vi "UHR-Fleezers Control (fpga) - 11.3h-g.vi"() -> ()   [LabVIEW 2012]
doc: "UHR-Fleezers Instrument Control Code (fpga)"
uses:
  <vilib>/Platform/TimedLoop/XDataNode/timing_clust.ctl
  <vilib>/Platform/TimedLoop/XDataNode/nitl_modes.ctl
  <vilib>/Platform/TimedLoop/XDataNode/wakeup.ctl
  <vilib>/rvi/eio/common/nirviEmuTemplateMethod_errors.vi
  <vilib>/rvi/interface/RandomDataEmulation/nirviRandomDataFPGAFIFO.vi
  <vilib>/rvi/interface/RandomDataEmulation/niFpgaRandomDataHandleErrors.vi
  <vilib>/rvi/Emulation/niFpgaSctlEmulationGetInTimedLoop.vi
  <vilib>/rvi/Emulation/niFpgaSctlEmulationGlobalWrite.vi
  <vilib>/rvi/Emulation/niFpgaSctlEmulationRegisterWithScheduler.vi
  <vilib>/rvi/Emulation/niFpgaSctlEmulationScheduler.vi
  <vilib>/Platform/TimedLoop/XDataNode/XDataNode.xnode
  <vilib>/eio/EIOMethodNode/EIOMethodNode.xnode
  <vilib>/eio/EIONode/EIONode.xnode
  <vilib>/rvi/DataTransferAndStorage/Container/XNode/niFpgaContainer.xnode
  <vilib>/rvi/interface/RandomDataEmulation/nirviRandomDataFpgaReadWriteTemplate.vi
  <vilib>/addons/control/pid/fpga.llb/XNode/niFpgaPID.xnode
  <vilib>/Platform/TimedLoop/XDataNode/XDNodeRunTimeDep.lvlib
panel:
  in  "Tab Control":T1(tab)=enum."Force FB"
  in  "Set 3":bool
  in  "Set 2":bool=TRUE
  in  "Set 1":bool=TRUE
  in  "Trap Pos to FIFO":bool
  in  "N of AI1 Int Acq Sets":i16=2 min=1 max=3 step=1
  out "AI Late Counter":u8
  in  "ai count":u16=400
  in  "+ phase":bool
  in  "Phase count adjustment":i16
  out "Relative phase":i16
  in  "AI to FIFO":bool
  out "BD1 Frequency Out 1":u64
  out "BD1 Frequency Out 2":u64
  out "Trap Pos FIFO Timeout":u16
  out "Trap AI FIFO Timeout":u16
  in  "Trap FIFO Set Timeout":i32
  in  "Tab Control 2":T2(tab)
  in  "RD":bool
  in  "FB1 output high":i16=3000
  in  "FB1 output low":i16
  in  "D1":i16
  in  "I1":i16=5
  in  "P1":i16=10
  in  "Swap F1 and F2":bool
  in  "Cont. Scan":bool
  in  "Abort scan":bool
  in  "Cycles per step":u64
  in  "Scan BD":bool
  in  "Number of scans":u16
  in  "Scan steps":u64
  in  "Scan freq.  increment":i64
  out "Scanning":bool
  in  "Start scan":bool
  in  "OSK Bd 1":bool
  in  "Reset Bd 1":bool
  in  "PMODE":bool
  in  "Direct RF Box \nCommunication":bool
  in  "Data BD 2":u8 format="%08b"
  in  "Data BD 1":u8 format="%08b"
  in  "Address":u8 format="%02x"
  in  "Update Data":bool
  in  "FPGA Controls\n RF Box":bool
  in  "Number Interlace Cycles":u8=2 min=1 max=3
  in  "Interlace Off Parameters":u8=1 min=1 max=3
  in  "Interlace ON/OFF":bool
  out "DIO Relative phase":i16
  in  "Phase count adjustment (DIO)":i16
  in  "+ phase (DIO)":bool
  out "DIO Late Counter":u8
  in  "DIO count 1 (ticks)":u16=400
  in  "DIO count 2 (ticks)":u16=400
  in  "DIO count 3 (ticks)":u16=400
  out "AI2 Y Sum Set 2":i16
  out "AI2 Y Sum Set 1":i16
  in  "FB Setpoint Set 1":i16 min=0 step=1
  in  "FB Reset Set 1":bool
  in  "FB On/Off Set 1":bool
  in  "FB Reset Set 2":bool
  in  "FB On/Off Set 2":bool
  in  "FB Setpoint Set 2":i16 min=0 step=1
  out "Scan I":u64
  in  "Amp switch delay":u16=5
  in  "BD 2 Amplitude 1":u16
  in  "BD 1 Amplitude 1":u16
  in  "BD 2 Frequency 1":u64
  in  "BD 1 Frequency 1":u64
  in  "BD 2 Amplitude 2":u16
  in  "BD 1 Amplitude 2":u16
  in  "BD 2 Frequency 2":u64
  in  "BD 1 Frequency 2":u64
  in  "BD 2 Amplitude 3":u16
  in  "BD 1 Amplitude 3":u16
  in  "BD 2 Frequency 3":u64
  in  "BD 1 Frequency 3":u64
  in  "FB2 output high":fxp<+/-,16,1>=0.999969482421875
  in  "FB2 output low":fxp<+/-,16,1>=-1.0
  in  "P2":fxp<+/-,16,8> format="%.11g"
  in  "I2":fxp<+/-,16,8>=10.0 format="%.11g"
  in  "D2":fxp<+/-,16,8> format="%.11g"
  in  "Negate Diff?":bool
  in  "Diff FB Measurement?":bool
  in  "FB Trig Integrate":u32=1
  out "TTrig?":bool
  in  "TTrig Negate Pos":bool=TRUE
  out "Trap Pos FB Int Signal":fxp<+/-,24,9> format="%.18g"
  out "Trap Pos FB Int-Norm Signal":fxp<+/-,16,1> format="%.16g"
  in  "FPGA TTrig Thresh":i64
  in  "FPGA Trap Trig":bool
  out "Trap Pos FB Action":i64
  in  "Trap Pos. FB Offset Factor":i64
  in  "Trap Pos. FB Mult Factor":i64=2
  in  "Trap Pos. FB Reset":bool
  in  "Trap Pos FB Monitor T1 or T2":bool
  in  "AI1 X Scale":u16
  in  "Trap Pos FB Int Count":u16=100
  in  "Trap Pos FB Negate Action":bool
  out "AI1 X Set 2":fxp<+/-,16,1>
  out "AI1 X Set 1":fxp<+/-,16,1>
  in  "Trap Pos. FB SP":fxp<+/-,16,1>
  in  "Force feedback":bool
  out "TTrig Sig":i64
  out "TTrig Fin Thresh":i64
  in  "1D or 2D Scan?":bool
  in  "Abort scan (MCL)":bool
  in  "MCL Scan Axis":bool
  in  "Cont. Scan (MCL)":bool
  out "Scan I (MCL)":u64
  in  "Number of scans (MCL)":u16
  out "Scanning MCL":bool
  in  "Scan steps (MCL)":u64
  in  "Cycles per step (MCL)":u64
  in  "Scan freq.  increment (MCL)":i16
  in  "Start scan (MCL)":bool
  in  "AO2":i16
  in  "AO1":i16
  out "MCL Late Counter":u8
  in  "MCL count":u32=800
  out "MCL Relative Phase":i16
  in  "Phase count adjustment (MCL)":i16
  in  "+ phase (MCL)":bool
  out "APD3 out state":bool
  in  "APD Gate Operating Mode":u8 max=2 step=1
  in  "Invert APD Gate":bool
  in  "APD Gate OFF Count":u16=100
  in  "APD Gate ON Count":u16=300
  out "APD 1 Gate Late Counter":u8
  out "APD 1 Gate Relative Phase":i16
  in  "Phase count adjustment (APD 1 Gate)":i16
  in  "+ phase (APD 1 Gate)":bool
  out "APD 2 Counts 0":u32
  out "APD 2 Counts 1":u32
  out "APD 1 Counts 0":u32
  out "APD 1 Counts 1":u32
  out "APD1 out state":bool
  in  "APD AO scale factor":i16=1
  in  "APD to FIFO":bool
  in  "APD Acq Rate Count":u32=20000000
  out "APD Acq Late Counter":u8
  out "APD Acq Relative Phase":i16
  in  "Phase Count Adjustment (APD Acq)":i16
  in  "+ phase (APD Acq)":bool
  in  "Phase count adjustment (APD 2 Gate)":i16
  out "APD 2 Gate Late Counter":u8
  out "APD 2 Gate Relative Phase":i16
  in  "+ phase (APD 2 Gate)":bool
  out "APD2 out state":bool
  out "APD 3 Counts 0":u32
  out "APD 3 Counts 1":u32
  out "APD 3 Gate Late Counter":u8
  in  "Phase count adjustment (APD 3 Gate)":i16
  out "APD 3 Gate Relative Phase":i16
  in  "+ phase (APD 3 Gate)":bool
  in  "D3":i16
  in  "I3":i16=5
  in  "P3":i16=10
  in  "Green Filter Flipper":bool
  in  "Green FB Count":u16=1200
  out "Green Late Counter":u8
  out "Green FB Relative Phase":i16
  in  "Phase count adjustment (Green FB)":i16=10
  in  "+ phase (Green FB)":bool
  out "Green FB Sum":i16
  in  "Green int current ON count adj":u16=150
  in  "Current Out":u16=30000
  in  "Green FB On/Off":bool
  in  "Green FB Setpoint":i16=250 min=0 step=1
  in  "Green FB Reset":bool
  in  "Operating Mode 2":u8=2 max=2 step=1
  in  "Invert GI 2":bool
  in  "Green interlace OFF count 2":u16=900
  in  "Green interlace ON count 2":u16=300
  out "GI Late Counter 2":u8
  out "GI Relative phase 2":i16
  in  "Phase count adjustment (GI) 2":i16=20
  in  "+ phase (GI) 2":bool
  in  "Green interlace OFF count":u16=100
  out "GI Relative phase":i16
  in  "Phase count adjustment (GI)":i16
  in  "+ phase (GI)":bool
  in  "Green interlace ON count":u16=300
  out "GI Late Counter":u8
  in  "Invert GI":bool
  in  "Operating Mode":u8 max=2 step=1
  in  "+ phase (RI)":bool
  out "RI Relative phase":i16
  out "RI Late Counter":u8
  in  "Red interlace ON count":u16=300
  in  "Red interlace OFF count":u16=100
  in  "Invert RI":bool
  in  "Red Laser Operating Mode":u8 max=2 step=1
  in  "Phase count adjustment (RI)":i16
  out "Red FB Intensity":i16
  in  "RI Current Out":u16=30000
  in  "Red FB On/Off":bool
  in  "D4":i16
  in  "I4":i16=5
  in  "P4":i16=10
  in  "Red FB Setpoint":i16=250 min=0 step=1
  in  "Red FB Reset":bool
  in  "RI Operating Mode 2":u8=2 max=2 step=1
  in  "Invert RI 2":bool
  in  "Phase count adjustment (BI AO)":i16=20
  in  "Blue current ON count adj (AO)":u16=150
  in  "BI Current Out":i16=30000
  in  "Blue FB On/Off":bool
  in  "D5":i16
  in  "I5":i16=5
  in  "P5":i16=10
  in  "Blue FB Setpoint":i16=250 min=0 step=1
  in  "Blue FB Reset":bool
  in  "BI Operating Mode (AO)":u8=2 max=2 step=1
  in  "Invert BI (AO)":bool
  in  "Blue OFF count (AO)":u16=900
  in  "Blue ON count (AO)":u16=300
  out "BI Late Counter (AO)":u8
  out "BI Relative phase (AO)":i16
  in  "+ phase (BI AO)":bool
  in  "Phase count adjustment (BI D)":i16
  in  "Blue Laser Operating Mode (D)":u8 max=2 step=1
  in  "Invert BI (D)":bool
  in  "Blue interlace OFF count (D)":u16=100
  in  "Blue interlace ON count (D)":u16=300
  out "Blue Late Counter (D)":u8
  out "BI Relative phase (D)":i16
  in  "+ phase (BI D)":bool
  out "Blue Intensity":i16
  # "Only one of these can be on\nat a time:"
  # "Raster Scan AOD"
  # "1 (X)"
  # "2 (Y)"
  # "IR Intensity Feedback (RF BD 1)"
  # "FB Gains Set 1"
  # "FB output range 1"
  # "FB Triggering Excitation Laser"
  # "Trap Pos. FB Gains"
  # "Trap Pos. FB Range"
  # "AO1 (Y)"
  # "2D"
  # "1D"
  # "AO2 (X)"
  # "APD AO for aligning"
  # "Detection Loop"
  # "Green fluorescent laser digital gate interlacing loop"
  # "0 Forced ON\n1 Forced OFF\n2 Interlacing"
  # "Green FB Gains"
  # "Red fluorescent laser digital gate interlacing loop"
  # "Detection Loop"
  # "0 Forced ON\n1 Forced OFF\n2 Interlacing"
  # "Analog/FB Control Loop\n(Disabled)"
  # "Digital Control Loop"
  # "Blue laser intensity reading"
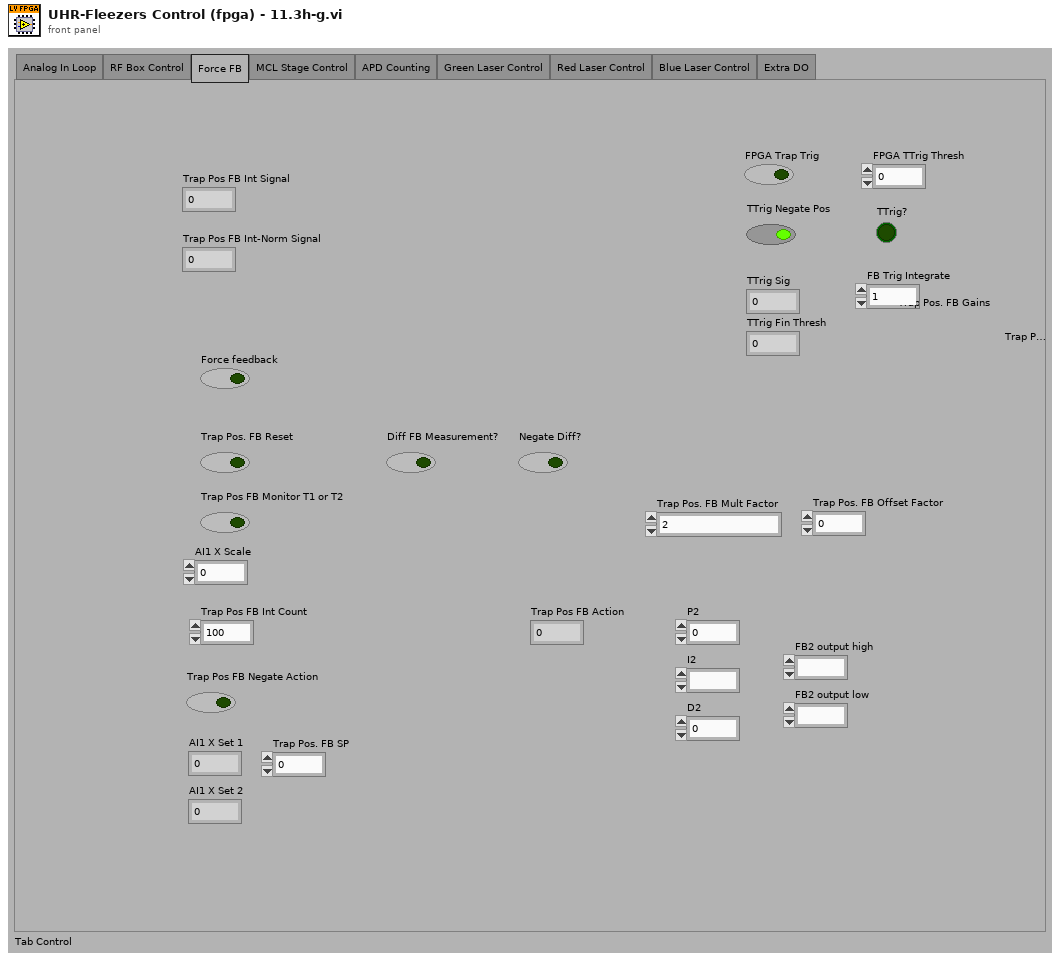
[diagram p1: front panel]
types:
  T1 = enum32{"Analog In Loop", "RF Box Control", "Force FB", "MCL Stage Control", "APD Counting", "Green Laser Control", "Red Laser Control", "Blue Laser Control", "Extra DO"}
  T2 = enum32{"Controls", "Interlacing Frequency and Amplitude Values"}
  T3 = typedef "XDNodeRunTimeDep.lvlib/timing_clust.ctl" = cluster{"Expected End [f-1]":u64, "Actual End [f-1]":u64, "Finished Late? [f-1]":bool, "Expected End [i-1]":u64, "Actual End [i-1]":u64, "Finished Late? [i-1]":bool, "Expected Start [i]":u64, "Actual Start [i]":u64, "Expected Start [f]":u64, "Actual Start [f]":u64, "Source Name":string, "Structure Name":string, "Period":i64, "Deadline":i64, "Offset":i64, "Start":i64, "Priority":i32, "Timeout":i32, "Mode":T4, "Wakeup Reason":T5, "Error":errorcluster, "Source Type":string, "Secondary Source Type":string, "Global End Time":u64, "Global Start Time":u64, "Frame Duration":u64, "Iteration Duration":u64, "Assigned CPU":i32, "I/O Scan Engine Mode":u32}
  T4 = typedef "XDNodeRunTimeDep.lvlib/nitl_modes.ctl" = enum32{"No Change", "Process missed periods, maintain original phase", "Discard missed periods, maintain original phase", "Process missed periods, ignore original phase", "Discard missed periods, ignore original phase"}
  T5 = typedef "XDNodeRunTimeDep.lvlib/wakeup.ctl" = enum32{"Normal", "Aborted", "Asynchronous wakeup", "Timing source error", "Timed loop error", "Timeout"}
  T6 = cluster{"proportional gain (Kc)":i16, "integral gain (Kc*Ts/Ti)":i16, "derivative gain (Kc*Td/Ts)":i16}
  T7 = cluster{"FB1 output high":i16, "FB1 output low":i16}
  T8 = cluster{"P2":fxp<+/-,16,8>, "I2":fxp<+/-,16,8>, "D2":fxp<+/-,16,8>}
  T9 = cluster{"FB2 output high":fxp<+/-,16,1>, "FB2 output low":fxp<+/-,16,1>}
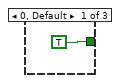
[diagram p3: hidden frame]
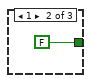
[diagram p4: hidden frame]
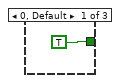
[diagram p5: hidden frame]
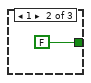
[diagram p6: hidden frame]
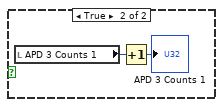
[diagram p7: hidden frame]
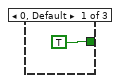
[diagram p8: hidden frame]
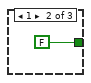
[diagram p9: hidden frame]
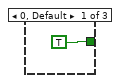
[diagram p10: hidden frame]
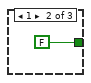
[diagram p11: hidden frame]
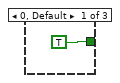
[diagram p12: hidden frame]
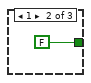
[diagram p13: hidden frame]
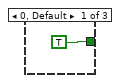
[diagram p14: hidden frame]
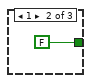
[diagram p15: hidden frame]
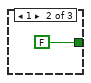
[diagram p18: hidden frame]
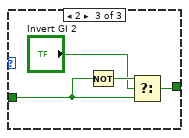
[diagram p19: hidden frame]
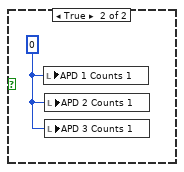
[diagram p20: hidden frame]
diagram:
  w3 = u16 0
  w5 = FALSE
  w2 = FALSE
  # "timing array current index"
  # "timing array"
  # "timing counter (phase adjusted here)"
  # "late counter"
  n1 = flat-sequence "FPGA initialization to do before running any of the loops" {
    tunnel: [u16 0 ("DIO count 3 (ticks)")] -> w1
    tunnel: [w12] -> _
    frame #0 {
      # "Start up expansion chassis early\nto avoid delays later"
      # "This pin controls udclk on the RF boards.\nWhen initially configuring the boards, this pin needs to be\nconfigured as a high impedance input.  Later it will be switched\nto an output."
      # "Initial setting of DIO data and \naddress to low (before reset).  \nThis needs to happen before the other\ncontrol method loops execute."
      n2 = xnode "FPGA I/O Node"("Chassis2/Mod4/AO0"=u16 0) -> ("Chassis2/Mod1/AI0"=w12:i16)  [unwired: 2 in, 2 out]
      n3 = xnode "FPGA I/O Method Node"("Enable"=FALSE) -> ()  [unwired: 1 in, 1 out]
      n4 = xnode "FPGA I/O Node"("Connector1/DIO0"=FALSE, "Connector1/DIO1"=FALSE, "Connector1/DIO2"=FALSE, "Connector1/DIO3"=FALSE, "Connector1/DIO4"=FALSE, "Connector1/DIO5"=FALSE, "Connector1/DIO6"=FALSE, "Connector1/DIO7"=FALSE, "Connector1/DIO8"=FALSE, "Connector1/DIO9"=FALSE, "Connector1/DIO10"=FALSE, "Connector1/DIO11"=FALSE, "Connector1/DIO12"=FALSE, "Connector1/DIO13"=FALSE, "Connector1/DIO15"=FALSE, "Connector1/DIO20"=FALSE, "Connector1/DIO21"=FALSE, "Connector1/DIO22"=FALSE, "Connector1/DIO23"=FALSE, "Connector1/DIO24"=FALSE, "Connector1/DIO25"=FALSE, "Connector1/DIO26"=FALSE, "Connector1/DIO27"=FALSE, "Connector1/DIO14"=FALSE) -> ()  [unwired: 24 in, 24 out]
    }
  }
  n5 = local read "AO1"() -> (w10:i16)
  n6 = local read "AO2"() -> (w9:i16)
  n7 = node-c288() -> (w8:T3)  [unwired: 1 in]
  n8 = timed-loop "RF box board DIO control: control bits" {
    timing: w8 -> [_]
    timing-out: [_] -> w7
    tunnel: [w42] -> _
    tunnel: w1 -> [w42]
    stop <- FALSE stop-if-true
    n9 = xnode "FPGA I/O Node"("Connector1/DIO16"="RD", "Connector1/DIO17"="PMODE", "Connector1/DIO18"="OSK Bd 1", "Connector1/DIO19"="Reset Bd 1", "Connector0/DIO3"="Green Filter Flipper") -> ()  [unwired: 5 in, 5 out]
  }
  n10 = while "RF box board DIO control: parallel communication" {
    shift-right: [w55] -> _
    shift-left: w1 -> [w54]
    shift-right: [w53] -> _
    shift-left: FALSE ("Swap F1 and F2") -> [w52]
    stop <- FALSE stop-if-true
    n11 = flat-sequence {
      tunnel: w52 -> [w59]
      tunnel: w54 -> [w57]
      tunnel: [w59] -> w51
      tunnel: [w58] -> w50
      tunnel: [w57] -> w49
      tunnel: [w65] -> w55
      tunnel: [w64] -> w53
      tunnel: w51 -> [w63]
      tunnel: w50 -> [w61]
      tunnel: w49 -> [w60]
      frame #0 {
        n12 = call "Loop Timer"("Count(Ticks)"=w57) -> ("Tick Count(Ticks)"=w58:u16)
      }
      frame #1 {
        n13 = flat-sequence {
          tunnel: ["FPGA Controls\n RF Box"] -> w62
          tunnel: w63 -> [w66]
          tunnel: [w106] -> w65
          tunnel: [w119] -> w64
          tunnel: w62 -> [w118]
          tunnel: w61 -> [w112]
          tunnel: w60 -> [w109]
          frame #0 {
            n14 = case shown="True" "FPGA Controls\n RF Box" {
              tunnel: w66 -> [_ w68]
              frame False {
              }
              frame True {
                n15 = flat-sequence {
                  tunnel: w68 -> [w74]
                  frame #0 {
                    n16 = First Call?() -> (First Call?: T/F=w69:bool)
                    n17 = case shown="True" w69 {
                      frame False {
                      }
                      frame True {
                        # "If first time data updated, be sure to set WR high and UDCLK low\nbefore setting data and address bits."
                        n18 = xnode "FPGA I/O Method Node"("Enable"=TRUE) -> ("FPGA I/O Out"=w71:refnum<k21>)  [unwired: 1 in]
                        n19 = xnode "FPGA I/O Node"("Connector1/DIO15"=TRUE) -> ()  [unwired: 1 in, 1 out]
                        n20 = xnode "FPGA I/O Node"("I/O Item"=FALSE ("Connector1/DIO30"), "FPGA I/O In"=w71) -> ()  [unwired: 1 out]
                      }
                    }
                  }
                  frame #1 {
                    n21 = flat-sequence {
                      tunnel: w74 -> [w75]
                      frame #0 {
                        # "switch frequency"
                        n22 = xnode "FPGA I/O Node"("Connector1/DIO36"=w75) -> ()  [unwired: 1 in, 1 out]
                      }
                      frame #1 {
                        n23 = call "Wait4"("Count(Ticks)"="Amp switch delay") -> ()  [unwired: 1 out]
                      }
                      frame #2 {
                        # "switch amplitude"
                        # "send udclk high"
                        n24 = xnode "FPGA I/O Node"("Connector1/DIO30"=TRUE ("Connector1/DIO15")) -> ()  [unwired: 1 in, 1 out]
                      }
                      frame #3 {
                        # "send udclk low"
                        n25 = xnode "FPGA I/O Node"("Connector1/DIO30"=FALSE ("Connector1/DIO15")) -> ()  [unwired: 1 in, 1 out]
                      }
                    }
                  }
                }
              }
            }
          }
          frame #1 {
            # "This is the prior cycle's on time"
            # "increment timing\nindex, reset to 0 if \nend of matrix"
            # "Reset to begginning (1) when number of cycles reached."
            # "timing index"
            # "build byte stacks for writing data\n(must correspond to addresses array constant)"
            # "Timing housekeeping"
            # "Adjust phase if late\n(maintains constant phase relationship between cycles)"
            n26 = Bundle("FB1 output high"="FB1 output high", "FB1 output low"="FB1 output low") -> (w79:T7)  [unwired: 1 in]
            n27 = Bundle("P1"="P1", "I1"="I1", "D1"="D1") -> (w80:cluster{"P1":i16, "I1":i16, "D1":i16})  [unwired: 1 in]
            n28 = feedback #1(u8 0 ("t")) -> (w115:u8)
            n29 = Increment(x=w115) -> (x+1=w159:u8)
            n30 = Increment(x="Number Interlace Cycles") -> (x+1=w154:u8)
            n31 = Equal?(x=w159, y=w154) -> (x = y?=w161:bool)
            n32 = Select(t=u8 1, s=w161, f=w159) -> (s? t:f=w114:u8)
            n33 = feedback-in #1(w114) -> ()
            n34 = Increment(x=w114) -> (x+1=w156:u8)
            n35 = Equal?(x=w156, y=w154) -> (x = y?=w157:bool)
            n36 = Select(t=u8 1, s=w157, f=w156) -> (s? t:f=w153:u8)
            n37 = Select(t=w153, s="Interlace ON/OFF", f="Interlace Off Parameters") -> (s? t:f=w137:u8)
            n38 = case shown="1, Default" w137 {
              tunnel: [w233 "BD 1 Frequency 2" "BD 1 Frequency 3"] -> w149
              tunnel: [w232 "BD 2 Frequency 2" "BD 2 Frequency 3"] -> w138
              tunnel: ["BD 2 Amplitude 1" "BD 2 Amplitude 2" "BD 2 Amplitude 3"] -> w94
              tunnel: [w221 w392 "BD 1 Amplitude 3"] -> w97
              tunnel: w80 -> [w195 w389 _]
              tunnel: w79 -> [w196 w388 _]
              frame 1, Default {
                w212 = fxp<+/-,24,9> 0.0 ("AI1 X Set 2")
                w205 = u16 0
                w228 = u64 0 ("f")
                # "This signal integration happens no matter what\nso that correct setpoints can be chosen before \nturning on the FB."
                # "Trap 1"
                n39 = local read "AI1 X Set 2"() -> (w208:fxp<+/-,16,1>)
                n40 = local read "AI1 X Set 1"() -> (w209:fxp<+/-,16,1>)
                n41 = local read "Scanning"() -> (w234:bool)
                n42 = Or(x=w234, y="Start scan") -> (x .or. y?=w226:bool)
                n43 = case shown="False" "Diff FB Measurement?" {
                  tunnel: w208 -> [w242 w251]
                  tunnel: w209 -> [w241 w252]
                  tunnel: [w239 w243] -> w210
                  frame False {
                    n44 = Select(t=w241, s="Trap Pos FB Monitor T1 or T2", f=w242) -> (s? t:f=w239:fxp<+/-,16,1>)
                  }
                  frame True {
                    n45 = Subtract(x=w252, y=w251) -> (x-y=w244:fxp<+/-,17,2>)
                    n46 = Not(x="Negate Diff?") -> (.not. x?=w250:bool)
                    n47 = Boolean To (0,1)(Boolean="Negate Diff?") -> (0, 1=w248:i16)
                    n48 = Boolean To (0,1)(Boolean=w250) -> (0, 1=w249:i16)
                    n49 = Negate(x=w248) -> (-x=w247:i16)
                    n50 = Add(x=w247, y=w249) -> (x+y=w245:i16)
                    n51 = Multiply(x=w245, y=w244) -> (x*y=w243:fxp<+/-,32,17>)
                  }
                }
                n52 = Not(x="Abort scan") -> (.not. x?=w224:bool)
                n53 = And(x=w224, y=w226) -> (x .and. y?=w223:bool)
                n54 = case "For raster scanning" shown="True" w223 {
                  tunnel: [u64 0 w378] -> w229
                  tunnel: "Start scan" -> [_ w363]
                  frame False {
                    n55 = local write "Scanning"(FALSE ("scanning")) -> ()
                  }
                  frame True {
                    w347 = i64 0
                    w346 = u64 0
                    # "scan incr."
                    # "freq. incr. mult."
                    # "count steps"
                    # "count number of cycles"
                    n56 = feedback #2(w346) -> (w375:u64)
                    n57 = Select(t=w346, s=w363, f=w375) -> (s? t:f=w377:u64)
                    n58 = Increment(x=w377) -> (x+1=w374:u64)
                    n59 = Greater?(x="Cycles per step", y=w374) -> (0:w356:bool)
                    n60 = Select(t=w374, s=w356, f=w346) -> (s? t:f=w373:u64)
                    n61 = feedback-in #2(w373) -> ()
                    n62 = feedback #3(w346) -> (w372:u64)
                    n63 = Select(t=w346, s=w363, f=w372) -> (s? t:f=w367:u64)
                    n64 = Increment(x=w367) -> (x+1=w371:u64)
                    n65 = Add(x="Scan steps", y="Scan steps") -> (x+y=w370:u64)
                    n66 = Select(t=w367, s=w356, f=w371) -> (s? t:f=w351:u64)
                    n67 = Greater?(x=w370, y=w351) -> (0:w350:bool)
                    n68 = Select(t=w351, s=w350, f=w346) -> (s? t:f=w368:u64)
                    n69 = feedback-in #3(w368) -> ()
                    n70 = Equal?(x="Scan steps", y=w351) -> (x = y?=w355:bool)
                    n71 = Greater?(x="Scan steps", y=w367) -> (0:w366:bool)
                    n72 = feedback #4(w347) -> (w369:i64)
                    n73 = Select(t=w347, s=w363, f=w369) -> (s? t:f=w353:i64)
                    n74 = Increment(x=w353) -> (x+1=w365:i64)
                    n75 = Decrement(x=w353) -> (x-1=w364:i64)
                    n76 = Select(t=w365, s=w366, f=w364) -> (s? t:f=w354:i64)
                    n77 = Select(t=w353, s=w355, f=w354) -> (s? t:f=w352:i64)
                    n78 = Select(t=w353, s=w356, f=w352) -> (s? t:f=w348:i64)
                    n79 = Select(t=w348, s=w350, f=w347) -> (s? t:f=w349:i64)
                    n80 = feedback-in #4(w349) -> ()
                    n81 = feedback #5(w346) -> (w362:u64)
                    n82 = Select(t=w346, s=w363, f=w362) -> (s? t:f=w358:u64)
                    n83 = Increment(x=w358) -> (x+1=w359:u64)
                    n84 = Select(t=w358, s=w350, f=w359) -> (s? t:f=w357:u64)
                    n85 = Greater?(x="Number of scans", y=w357) -> (0:w343:bool)
                    n86 = Multiply(x="Scan freq.  increment", y=w353) -> (x*y=w378:i64)
                    n87 = Select(t=TRUE, s="Cont. Scan", f=w343) -> (s? t:f=w342:bool)
                    "Scanning" <- w342
                    n88 = Select(t=w357, s=w342, f=w346) -> (s? t:f=w360:u64)
                    n89 = feedback-in #5(w360) -> ()
                    n90 = Increment(x=w357) -> (x+1=→"Scan I":u64)
                  }
                }
                n91 = feedback #6(w205) -> (w204:u16)
                n92 = Increment(x=w204) -> (x+1=w206:u16)
                n93 = Greater Or Equal?(x=w206, y="Trap Pos FB Int Count") -> (x >= y?=w197:bool)
                n94 = Select(t=w205, s=w197, f=w206) -> (s? t:f=w207:u16)
                n95 = feedback-in #6(w207) -> ()
                n96 = feedback #7(w212) -> (w211:fxp<+/-,24,9>)
                n97 = Add(x=w210, y=w211) -> (x+y=w203:fxp<+/-,24,9>)
                n98 = case "For intensity feedback" shown="True" "FB On/Off Set 1" {
                  tunnel: "BD 1 Amplitude 1" -> [w380 _]
                  tunnel: [w380 w384] -> w221
                  tunnel: w196 -> [_ w381]
                  tunnel: w195 -> [_ w382]
                  frame False {
                  }
                  frame True {
                    n99 = local read "AI2 Y Sum Set 1"() -> (w385:i16)
                    n100 = call "Slower PID.vi"("process variable"=w385, "reset?"="FB Reset Set 1", "setpoint"="FB Setpoint Set 1", "PID gains (x 2^8)"=w382, "output range"=w381) -> ("output"=w386:i16)  [unwired: 10 out]
                    n101 = To Unsigned Word Integer(number=w386) -> (unsigned 16bit integer=w384:u16)
                  }
                }
                n102 = Select(t=w212, s=w197, f=w203) -> (s? t:f=w215:fxp<+/-,24,9>)
                n103 = feedback-in #7(w215) -> ()
                n104 = Divide(x=w203, y="Trap Pos FB Int Count") -> (x/y=w198:fxp<+/-,16,1>)
                n105 = feedback #8(fxp<+/-,24,9> 0.0 ("AI1 X Set 2")) -> (w216:fxp<+/-,24,9>)
                n106 = Select(t=w203, s=w197, f=w216) -> (s? t:f=w217:fxp<+/-,24,9>)
                "Trap Pos FB Int Signal" <- w217
                n107 = feedback-in #8(w217) -> ()
                n108 = feedback #9(fxp<+/-,16,1> 0.0 ("Trap Pos FB Int-Norm Signal")) -> (w200:fxp<+/-,16,1>)
                n109 = Select(t=w198, s=w197, f=w200) -> (s? t:f=w199:fxp<+/-,16,1>)
                "Trap Pos FB Int-Norm Signal" <- w199
                n110 = feedback-in #9(w199) -> ()
                n111 = case "For position feedback" shown="True" "Force feedback" {
                  tunnel: [i64 0 w258] -> w218
                  tunnel: w198 -> [_ w255]
                  tunnel: w197 -> [_ w254]
                  frame False {
                  }
                  frame True {
                    n112 = feedback #10(i64 0) -> (w257:i64)
                    n113 = case shown="True" w254 {
                      tunnel: [w259 w273] -> w258
                      tunnel: w257 -> [w259 _]
                      tunnel: w255 -> [_ w267]
                      frame False {
                      }
                      frame True {
                        w277 = u32 0
                        n114 = Bundle("P2"="P2", "I2"="I2", "D2"="D2") -> (w263:T8)  [unwired: 1 in]
                        n115 = Bundle("FB2 output high"="FB2 output high", "FB2 output low"="FB2 output low") -> (w260:T9)  [unwired: 1 in]
                        n116 = xnode ("PID")("process variable"=w267, "reset?"="Trap Pos. FB Reset", "setpoint"="Trap Pos. FB SP", "PID gains"=w263, "output range"=w260) -> ("output"=w289:fxp<+/-,16,1>)
                        n117 = Negate(x=w289) -> (-x=w288:fxp<+/-,17,2>)
                        n118 = Select(t=w288, s="Trap Pos FB Negate Action", f=w289) -> (s? t:f=w285:fxp<+/-,17,2>)
                        n119 = Scale By Power Of 2(n=u32 15, x=u32 1) -> (x*2^n=w282:u32)
                        n120 = Multiply(x=w285, y=w282) -> (x*y=w281:fxp<+/-,17,17>)
                        n121 = To Quad Integer(1:w281) -> (0:w293:i64)
                        "Trap Pos FB Action" <- w293
                        n122 = Multiply(x=w293, y="Trap Pos. FB Mult Factor") -> (x*y=w291:i64)
                        n123 = Add(x=w291, y="Trap Pos. FB Offset Factor") -> (x+y=w273:i64)
                        n124 = feedback #11() -> (w274:i64)  [unwired: 1 in]
                        n125 = Add(x=w273, y=w274) -> (x+y=w271:i64)
                        n126 = feedback #12(w277) -> (w279:u32)
                        n127 = Increment(x=w279) -> (x+1=w268:u32)
                        n128 = Greater Or Equal?(x=w268, y="FB Trig Integrate") -> (x >= y?=w269:bool)
                        n129 = Select(t=i64 0, s=w269, f=w271) -> (s? t:f=w275:i64)
                        n130 = feedback-in #11(w275) -> ()
                        n131 = Select(t=w277, s=w269, f=w268) -> (s? t:f=w278:u32)
                        n132 = feedback-in #12(w278) -> ()
                        n133 = And(x=w269, y="FPGA Trap Trig") -> (x .and. y?=w276:bool)
                        n134 = case "Trap FB trigger excitation laser ON" shown="True" w276 {
                          tunnel: w271 -> [_ w297]
                          tunnel: w268 -> [_ w295]
                          frame False {
                          }
                          frame True {
                            n135 = Not(x="TTrig Negate Pos") -> (.not. x?=w304:bool)
                            n136 = Boolean To (0,1)(Boolean="TTrig Negate Pos") -> (0, 1=w302:i16)
                            n137 = Boolean To (0,1)(Boolean=w304) -> (0, 1=w303:i16)
                            n138 = Negate(x=w302) -> (-x=w301:i16)
                            n139 = Add(x=w301, y=w303) -> (x+y=w300:i16)
                            n140 = Multiply(x=w300, y=w297) -> (x*y=w299:i64)
                            "TTrig Sig" <- w299
                            n141 = Multiply(x="FPGA TTrig Thresh", y=w295) -> (x*y=w296:i64)
                            "TTrig Fin Thresh" <- w296
                            n142 = Greater Or Equal?(x=w299, y=w296) -> (x >= y?=w298:bool)
                            n143 = case shown="True" w298 {
                              frame False {
                              }
                              frame True {
                                w307 = TRUE ("Green FB On/Off")
                                w309 = u8 2 ("Operating Mode")
                                n144 = local write "Operating Mode 2"(w309) -> ()
                                n145 = local write "Operating Mode"(w309) -> ()
                                n146 = local write "Green FB On/Off"(w307) -> ()
                                n147 = local write "FPGA Trap Trig"(FALSE ("FPGA Trap Trig")) -> ()
                                "TTrig?" <- w307
                              }
                            }
                          }
                        }
                      }
                    }
                    n148 = feedback-in #10(w258) -> ()
                  }
                }
                n149 = Select(t=w228, s="Scan BD", f=w229) -> (s? t:f=w227:u64)
                n150 = Select(t=w229, s="Scan BD", f=w228) -> (s? t:f=w230:u64)
                n151 = Add(x=w227, y="BD 2 Frequency 1") -> (x+y=w232:u64)
                n152 = Compound Arithmetic op=ADD("BD 1 Frequency 1", w218, w230) -> (w233:u64)
                "BD1 Frequency Out 1" <- w233
              }
              frame 2 {
                # "Trap 2"
                n153 = case shown="True" "FB On/Off Set 2" {
                  tunnel: [w396 w399] -> w392
                  tunnel: "BD 1 Amplitude 2" -> [w396 _]
                  tunnel: w389 -> [_ w398]
                  tunnel: w388 -> [_ w397]
                  frame False {
                  }
                  frame True {
                    n154 = local read "AI2 Y Sum Set 2"() -> (w402:i16)
                    n155 = call "Slower PID.vi"("process variable"=w402, "reset?"="FB Reset Set 2", "setpoint"="FB Setpoint Set 2", "PID gains (x 2^8)"=w398, "output range"=w397) -> ("output"=w400:i16)  [unwired: 10 out]
                    n156 = To Unsigned Word Integer(number=w400) -> (unsigned 16bit integer=w399:u16)
                  }
                }
                "BD1 Frequency Out 2" <- "BD 1 Frequency 2"
              }
              frame 3 {
                # "Fluorescence period"
              }
            }
            n157 = feedback-in #13(w112) -> ()
            n158 = feedback #13(w112) -> (w111:u16)
            n159 = Select(t=w114, s="Interlace ON/OFF", f="Interlace Off Parameters") -> (s? t:f=w152:u8)
            n160 = Subtract(x=w112, y=w111) -> (x-y=w110:u16)
            n161 = Subtract "The error"(x=w110, y=w109) -> (x-y=w87:u16)
            n162 = case shown="1, Default" w152 {
              tunnel: ["DIO count 1 (ticks)" "DIO count 2 (ticks)" "DIO count 3 (ticks)"] -> w108
              frame 1, Default {
              }
              frame 2 {
              }
              frame 3 {
              }
            }
            n163 = Number To Boolean Array(number=w87) -> (Boolean array=w88:bool[])
            n164 = Or Array Elements(Boolean array=w88) -> (logical OR=w86:bool)
            n165 = Boolean To (0,1)(Boolean=w86) -> (0, 1=w93:i16)
            n166 = To Unsigned Byte Integer(number=w93) -> (unsigned 8bit integer=w90:u8)
            n167 = feedback #14(u8 0) -> (w91:u8)
            n168 = Add(x=w90, y=w91) -> (x+y=w89:u8)
            "DIO Late Counter" <- w89
            n169 = feedback-in #14(w89) -> ()
            n170 = Subtract(x=w108, y=w87) -> (x-y=w107:u16)
            n171 = Split Number(x=w149) -> (hi(x)=w148:u32, lo(x)=w147:u32)
            n172 = Split Number(x=w138) -> (hi(x)=w143:u32, lo(x)=w142:u32)
            n173 = Boolean To (0,1)(Boolean="+ phase (DIO)") -> (0, 1=w104:i16)
            n174 = Split Number(x=w148) -> (lo(x)=w146:u16)  [unwired: 1 out]
            n175 = Split Number(x=w147) -> (hi(x)=w145:u16, lo(x)=w144:u16)
            n176 = Split Number(x=w143) -> (lo(x)=w141:u16)  [unwired: 1 out]
            n177 = Split Number(x=w142) -> (hi(x)=w140:u16, lo(x)=w139:u16)
            n178 = Split Number(x=w97) -> (hi(x)=w99:u8, lo(x)=w98:u8)
            n179 = Split Number(x=w94) -> (hi(x)=w96:u8, lo(x)=w95:u8)
            n180 = Split Number(x=w146) -> (hi(x)=w136:u8, lo(x)=w135:u8)
            n181 = Split Number(x=w145) -> (hi(x)=w134:u8, lo(x)=w133:u8)
            n182 = Split Number(x=w141) -> (hi(x)=w129:u8, lo(x)=w128:u8)
            n183 = Split Number(x=w144) -> (hi(x)=w132:u8, lo(x)=w131:u8)
            n184 = Split Number(x=w140) -> (hi(x)=w127:u8, lo(x)=w126:u8)
            n185 = Split Number(x=w139) -> (hi(x)=w125:u8, lo(x)=w124:u8)
            n186 = Multiply(x=w104, y="Phase count adjustment (DIO)") -> (x*y=w100:i16)
            n187 = feedback #15(i16 0) -> (w102:i16)
            n188 = Subtract(x=w102, y=w100) -> (x-y=w101:i16)
            "DIO Relative phase" <- w101
            n189 = feedback-in #15(w101) -> ()
            n190 = Add(x=w107, y=w100) -> (x+y=w106:u16)
            n191 = Build Array "BD 1 A Stack"(w99, w98) -> (w121:u8[])
            n192 = Build Array "BD 2 A Stack"(w96, w95) -> (w120:u8[])
            n193 = Build Array "BD 1 nu Stack"(w136, w135, w134, w133, w132, w131) -> (w130:u8[])
            n194 = Build Array "BD 2 nu Stack"(w129, w128, w127, w126, w125, w124) -> (w123:u8[])
            n195 = case shown="2" w137 {
              tunnel: [w187 w190] -> w119
              tunnel: [u8 10 u8 4] -> w122
              tunnel: "Swap F1 and F2" -> [w188 w190]
              frame 2 {
                # "F2"
                n196 = Not(x=w188) -> (.not. x?=w187:bool)
              }
              frame 1, Default {
                # "low chooses F1"
                # "F1"
              }
            }
            n197 = case "If FPGA is controlling (toggling) RF synth" shown="True" w118 {
              tunnel: w130 -> [_ w166]
              tunnel: w123 -> [_ w165]
              tunnel: w122 -> [_ w164]
              tunnel: w121 -> [_ w163]
              tunnel: w120 -> [_ w162]
              frame False {
              }
              frame True {
                # "Write next amp.\n(wait until beginning of next loop iteration to update)"
                n198 = flat-sequence "Update the next F1 and F2 frequency value (the actual frequency won't change until FSK is switched).\nThen load the next amplitude value into buffer, but don't update it until the next cycle." {
                  tunnel: w166 -> [w169]
                  tunnel: w165 -> [w168]
                  tunnel: w164 -> [w167]
                  tunnel: w163 -> [w180]
                  tunnel: w162 -> [w179]
                  frame #0 {
                    n199 = for {
                      tunnel: w169 -> [w175] mode=indexing
                      tunnel: w168 -> [w174] mode=indexing
                      tunnel: w167 -> [w172]
                      i -> [w173]
                      # "Write next freq."
                      n200 = To Unsigned Byte Integer(number=w173) -> (unsigned 8bit integer=w170:u8)
                      n201 = Add(x=w172, y=w170) -> (x+y=w171:u8)
                      n202 = call "write to RF synth bd.vi"("Address Byte"=w171, "BD 2 Byte"=w174, "BD 1 Byte"=w175) -> ()
                    }
                  }
                  frame #1 {
                    # "send udclk high"
                    n203 = xnode "FPGA I/O Node"("Connector1/DIO30"=TRUE ("Connector1/DIO15")) -> ()  [unwired: 1 in, 1 out]
                  }
                  frame #2 {
                    n204 = xnode "FPGA I/O Node"("Connector1/DIO30"=FALSE ("Connector1/DIO15")) -> ()  [unwired: 1 in, 1 out]
                  }
                  frame #3 {
                    n205 = for {
                      tunnel: w180 -> [w186] mode=indexing
                      tunnel: w179 -> [w185] mode=indexing
                      tunnel: u8 33 -> [w183]
                      i -> [w184]
                      n206 = To Unsigned Byte Integer(number=w184) -> (unsigned 8bit integer=w181:u8)
                      n207 = Add(x=w183, y=w181) -> (x+y=w182:u8)
                      n208 = call "write to RF synth bd.vi"("Address Byte"=w182, "BD 2 Byte"=w185, "BD 1 Byte"=w186) -> ()
                    }
                  }
                }
              }
            }
          }
        }
      }
    }
  }
  n209 = while "RF box board direct communication loop" {
    tunnel: w1 -> [_]
    stop <- FALSE stop-if-true
    n210 = case "Whether to use direct communication method (only use one method at a time)" shown="True" "Direct RF Box \nCommunication" {
      frame False {
      }
      frame True {
        n211 = case shown="True" "Update Data" {
          frame False {
          }
          frame True {
            n212 = flat-sequence {
              frame #0 {
                n213 = First Call?() -> (First Call?: T/F=w411:bool)
                n214 = case shown="True" w411 {
                  frame False {
                  }
                  frame True {
                    # "If first time data updated, be sure to set WR high\nbefore setting data and address bits."
                    n215 = flat-sequence {
                      frame #0 {
                        n216 = xnode "FPGA I/O Node"("Connector1/DIO15"=TRUE) -> ()  [unwired: 1 in, 1 out]
                      }
                      frame #1 {
                        n217 = call "Wait"("Count(Ticks)"=u8 40 ("DO Delay 3 (Ticks)")) -> ()  [unwired: 1 out]
                      }
                    }
                  }
                }
              }
              frame #1 {
                n218 = Number To Boolean Array(number="Address") -> (Boolean array=w460:bool[])
                n219 = Number To Boolean Array(number="Data BD 1") -> (Boolean array=w461:bool[])
                n220 = Number To Boolean Array(number="Data BD 2") -> (Boolean array=w430:bool[])
                n221 = Index Array(array=w461, index=7) -> (element=w445:bool)
                n222 = Index Array(array=w461, index=6) -> (element=w444:bool)
                n223 = Index Array(array=w461, index=5) -> (element=w443:bool)
                n224 = Index Array(array=w461, index=4) -> (element=w442:bool)
                n225 = Index Array(array=w461, index=3) -> (element=w441:bool)
                n226 = Index Array(array=w461, index=2) -> (element=w440:bool)
                n227 = Index Array(array=w461, index=1) -> (element=w439:bool)
                n228 = Index Array(array=w461, index=0) -> (element=w438:bool)
                n229 = Index Array(array=w460, index=5) -> (element=w437:bool)
                n230 = Index Array(array=w460, index=4) -> (element=w436:bool)
                n231 = Index Array(array=w460, index=3) -> (element=w435:bool)
                n232 = Index Array(array=w460, index=2) -> (element=w434:bool)
                n233 = Index Array(array=w460, index=1) -> (element=w433:bool)
                n234 = Index Array(array=w460, index=0) -> (element=w432:bool)
                n235 = Index Array(array=w430, index=7) -> (element=w421:bool)
                n236 = Index Array(array=w430, index=6) -> (element=w420:bool)
                n237 = Index Array(array=w430, index=5) -> (element=w419:bool)
                n238 = Index Array(array=w430, index=4) -> (element=w418:bool)
                n239 = Index Array(array=w430, index=3) -> (element=w417:bool)
                n240 = Index Array(array=w430, index=2) -> (element=w416:bool)
                n241 = Index Array(array=w430, index=1) -> (element=w415:bool)
                n242 = Index Array(array=w430, index=0) -> (element=w414:bool)
                n243 = xnode "FPGA I/O Node"("Connector1/DIO0"=w445, "Connector1/DIO1"=w444, "Connector1/DIO2"=w443, "Connector1/DIO3"=w442, "Connector1/DIO4"=w441, "Connector1/DIO5"=w440, "Connector1/DIO6"=w439, "Connector1/DIO7"=w438, "Connector1/DIO8"=w437, "Connector1/DIO9"=w436, "Connector1/DIO10"=w435, "Connector1/DIO11"=w434, "Connector1/DIO12"=w433, "Connector1/DIO13"=w432, "Connector1/DIO20"=w421, "Connector1/DIO21"=w420, "Connector1/DIO22"=w419, "Connector1/DIO23"=w418, "Connector1/DIO24"=w417, "Connector1/DIO25"=w416, "Connector1/DIO26"=w415, "Connector1/DIO27"=w414) -> ()  [unwired: 22 in, 22 out]
              }
              frame #2 {
                # "wait and then apply write signal"
                n244 = call "Wait2"("Count(Ticks)"=u8 40 ("DO Delay 1 (Ticks)")) -> ()  [unwired: 1 out]
              }
              frame #3 {
                # "sending bit low writes data to board buffer"
                n245 = xnode "FPGA I/O Node"("Connector1/DIO15"=FALSE) -> ()  [unwired: 1 in, 1 out]
              }
              frame #4 {
                # "wait then return write signal"
                n246 = call "Wait3"("Count(Ticks)"=u8 40 ("DO Delay 2 (Ticks)")) -> ()  [unwired: 1 out]
              }
              frame #5 {
                # "sending bit high makes ready to\nwrite more data"
                n247 = xnode "FPGA I/O Node"("Connector1/DIO15"=TRUE) -> ()  [unwired: 1 in, 1 out]
              }
            }
          }
        }
      }
    }
  }
  n248 = To Unsigned Long Integer(number=w1) -> (unsigned 32bit integer=w6:u32)
  n249 = while "APD 1 Counter" {
    tunnel: w1 -> [_]
    stop <- FALSE stop-if-true
    n250 = flat-sequence {
      frame #0 {
        n251 = xnode "FPGA I/O Method Node"("FPGA I/O In"=refnum<k21> "Connector0/DIO0" ("APD 1 DO"), "Timeout"=-1) -> ()  [unwired: 2 out]
      }
      frame #1 {
        n252 = local read "APD1 out state"() -> (w471:bool)
        n253 = case shown="False" w471 {
          frame False {
            n254 = local read "APD 1 Counts 0"() -> (w473:u32)
            n255 = Increment(x=w473) -> (x+1=→"APD 1 Counts 0":u32)
          }
          frame True {
            n256 = local read "APD 1 Counts 1"() -> (w475:u32)
            n257 = Increment(x=w475) -> (x+1=→"APD 1 Counts 1":u32)
          }
        }
      }
    }
  }
  n258 = while "APD 2 Counter" {
    tunnel: w1 -> [_]
    stop <- FALSE stop-if-true
    n259 = flat-sequence {
      frame #0 {
        n260 = xnode "FPGA I/O Method Node"("FPGA I/O In"=refnum<k21> "Connector0/DIO1" ("APD 2 DO"), "Timeout"=-1) -> ()  [unwired: 2 out]
      }
      frame #1 {
        n261 = local read "APD2 out state"() -> (w479:bool)
        n262 = case shown="False" w479 {
          frame False {
            n263 = local read "APD 2 Counts 0"() -> (w481:u32)
            n264 = Increment(x=w481) -> (x+1=→"APD 2 Counts 0":u32)
          }
          frame True {
            n265 = local read "APD 2 Counts 1"() -> (w483:u32)
            n266 = Increment(x=w483) -> (x+1=→"APD 2 Counts 1":u32)
          }
        }
      }
    }
  }
  n267 = while "APD 2 Gating" {
    shift-right: [w487] -> _
    shift-left: w1 -> [w492]
    shift-right: [w486] -> _
    shift-left: w5 -> [w484]
    stop <- FALSE stop-if-true
    n268 = flat-sequence {
      tunnel: w492 -> [w495]
      tunnel: [w496] -> w490
      tunnel: [w495] -> w488
      tunnel: [w494] -> w485
      tunnel: w484 -> [w494]
      tunnel: [w499] -> w491
      tunnel: w490 -> [w499]
      tunnel: [w498] -> w489
      tunnel: w488 -> [w498]
      tunnel: w485 -> [w497]
      tunnel: [w517] -> w487
      tunnel: w491 -> [w528]
      tunnel: w489 -> [w526]
      tunnel: [w521] -> w486
      frame #0 {
        n269 = call "Loop Timer8"("Count(Ticks)"=w495) -> ("Tick Count(Ticks)"=w496:u16)
      }
      frame #1 {
        # "Signal is then sent through \na transistor before APD"
        n270 = xnode "FPGA I/O Node"("Connector0/DIO8"=w497) -> ()  [unwired: 1 in, 1 out]
      }
      frame #2 {
        n271 = local read "APD Gate ON Count"() -> (w510:u16)
        n272 = local read "APD Gate OFF Count"() -> (w509:u16)
        n273 = feedback #16(TRUE) -> (w523:bool)
        n274 = feedback-in #17(w528) -> ()
        n275 = feedback #17(w528) -> (w511:u16)
        n276 = Not(x=w523) -> (.not. x?=w520:bool)
        n277 = feedback-in #16(w520) -> ()
        n278 = Subtract(x=w528, y=w511) -> (x-y=w527:u16)
        n279 = Select(t=w510, s=w520, f=w509) -> (s? t:f=w525:u16)
        n280 = Subtract(x=w527, y=w526) -> (x-y=w502:u16)
        n281 = Subtract(x=w525, y=w502) -> (x-y=w516:u16)
        n282 = Number To Boolean Array(number=w502) -> (Boolean array=w501:bool[])
        n283 = Or Array Elements(Boolean array=w501) -> (logical OR=w500:bool)
        n284 = Boolean To (0,1)(Boolean="+ phase (APD 2 Gate)") -> (0, 1=w514:i16)
        n285 = Multiply(x=w514, y="Phase count adjustment (APD 2 Gate)") -> (x*y=w512:i16)
        n286 = Boolean To (0,1)(Boolean=w500) -> (0, 1=w507:i16)
        n287 = Add(x=w516, y=w512) -> (x+y=w517:u16)
        n288 = To Unsigned Byte Integer(number=w507) -> (unsigned 8bit integer=w504:u8)
        n289 = feedback #18(i16 0) -> (w519:i16)
        n290 = Subtract(x=w519, y=w512) -> (x-y=w518:i16)
        "APD 2 Gate Relative Phase" <- w518
        n291 = feedback-in #18(w518) -> ()
        n292 = feedback #19(u8 0) -> (w505:u8)
        n293 = Add(x=w504, y=w505) -> (x+y=w503:u8)
        "APD 2 Gate Late Counter" <- w503
        n294 = feedback-in #19(w503) -> ()
        n295 = local read "APD Gate Operating Mode"() -> (w508:u8)
        n296 = case shown="2" w508 {
          tunnel: [TRUE FALSE w534] -> w521
          tunnel: w523 -> [_ _ w532]
          frame 0, Default {
          }
          frame 1 {
          }
          frame 2 {
            n297 = local read "Invert APD Gate"() -> (w531:bool)
            n298 = Not(x=w532) -> (.not. x?=w533:bool)
            n299 = Select(t=w533, s=w531, f=w532) -> (s? t:f=w534:bool)
          }
        }
      }
    }
  }
  n300 = while "532 nm green fluorescent laser interlacing (DO to IA 532 nm AOM ME amp)." {
    shift-right: [w538] -> _
    shift-left: w1 -> [w543]
    shift-right: [w537] -> _
    shift-left: w2 -> [w535]
    stop <- FALSE stop-if-true
    n301 = flat-sequence {
      tunnel: w543 -> [w546]
      tunnel: [w547] -> w541
      tunnel: [w546] -> w539
      tunnel: [w545] -> w536
      tunnel: w535 -> [w545]
      tunnel: [w550] -> w542
      tunnel: w541 -> [w550]
      tunnel: [w549] -> w540
      tunnel: w539 -> [w549]
      tunnel: w536 -> [w548]
      tunnel: [w559] -> w538
      tunnel: w542 -> [w579]
      tunnel: w540 -> [w576]
      tunnel: [w568] -> w537
      frame #0 {
        n302 = call "Loop Timer4"("Count(Ticks)"=w546) -> ("Tick Count(Ticks)"=w547:u16)
      }
      frame #1 {
        # "Then to PRL 440 amp"
        n303 = xnode "FPGA I/O Node"("Connector1/DIO39"=w548) -> ()  [unwired: 1 in, 1 out]
      }
      frame #2 {
        n304 = feedback-in #20(w579) -> ()
        n305 = feedback #20(w579) -> (w578:u16)
        n306 = Subtract(x=w579, y=w578) -> (x-y=w577:u16)
        n307 = Subtract(x=w577, y=w576) -> (x-y=w552:u16)
        n308 = Number To Boolean Array(number=w552) -> (Boolean array=w553:bool[])
        n309 = Or Array Elements(Boolean array=w553) -> (logical OR=w551:bool)
        n310 = Boolean To (0,1)(Boolean="+ phase (GI)") -> (0, 1=w564:i16)
        n311 = Multiply(x=w564, y="Phase count adjustment (GI)") -> (x*y=w561:i16)
        n312 = Boolean To (0,1)(Boolean=w551) -> (0, 1=w558:i16)
        n313 = To Unsigned Byte Integer(number=w558) -> (unsigned 8bit integer=w555:u8)
        n314 = feedback #21(i16 0) -> (w562:i16)
        n315 = feedback #22(u8 0) -> (w556:u8)
        n316 = Add(x=w555, y=w556) -> (x+y=w554:u8)
        "GI Late Counter" <- w554
        n317 = feedback-in #22(w554) -> ()
        n318 = Subtract(x=w562, y=w561) -> (x-y=w560:i16)
        "GI Relative phase" <- w560
        n319 = feedback-in #21(w560) -> ()
        n320 = feedback #23(TRUE) -> (w571:bool)
        n321 = case shown="2" "Operating Mode" {
          tunnel: [TRUE FALSE w585] -> w568
          tunnel: w571 -> [_ _ w582]
          frame 0, Default {
          }
          frame 1 {
          }
          frame 2 {
            n322 = Not(x=w582) -> (.not. x?=w584:bool)
            n323 = Select(t=w584, s="Invert GI", f=w582) -> (s? t:f=w585:bool)
          }
        }
        n324 = Not(x=w571) -> (.not. x?=w567:bool)
        n325 = Select(t="Green interlace ON count", s=w567, f="Green interlace OFF count") -> (s? t:f=w573:u16)
        n326 = Subtract(x=w573, y=w552) -> (x-y=w565:u16)
        n327 = Add(x=w565, y=w561) -> (x+y=w559:u16)
        n328 = feedback-in #23(w567) -> ()
      }
    }
  }
  n329 = while "DAQ AI set 1" {
    shift-right: [w586] -> _
    shift-left: w1 -> [w591]
    stop <- FALSE stop-if-true
    n330 = flat-sequence {
      tunnel: w591 -> [w601]
      tunnel: [w602] -> w589
      tunnel: [w601] -> w588
      tunnel: [w612] -> w599
      tunnel: [w611] -> w598
      tunnel: [w610] -> w597
      tunnel: [w609] -> w596
      tunnel: [w608] -> w595
      tunnel: [w607] -> w594
      tunnel: [w606] -> w593
      tunnel: [w605] -> w592
      tunnel: [w604] -> w590
      tunnel: w589 -> [w604]
      tunnel: w588 -> [w603]
      tunnel: [w603] -> w587
      tunnel: [w641] -> w586
      tunnel: w599 -> [w668]
      tunnel: w598 -> [w633]
      tunnel: w597 -> [w634]
      tunnel: w596 -> [w667]
      tunnel: w595 -> [w657]
      tunnel: w594 -> [w656]
      tunnel: w593 -> [w655]
      tunnel: w592 -> [w654]
      tunnel: w590 -> [w651]
      tunnel: w587 -> [w648]
      frame #0 {
        n331 = call "Loop Timer3"("Count(Ticks)"=w601) -> ("Tick Count(Ticks)"=w602:u16)
      }
      frame #1 {
        n332 = xnode "FPGA I/O Node"("Connector1/DIO31"=TRUE ("Connector1/DIO33")) -> ("Connector0/AI0"=w612:i16, "Connector0/AI1"=w611:i16, "Connector0/AI2"=w610:i16, "Connector0/AI3"=w609:i16, "Connector0/AI4"=w608:i16, "Connector0/AI5"=w607:i16, "Connector0/AI6"=w606:i16, "Connector0/AI7"=w605:i16)  [unwired: 9 in, 9 out]
      }
      frame #2 {
        w637 = FALSE ("AI to FIFO")
        # "Adjust phase after data acquired if button pressed"
        n333 = feedback #24(i16 1) -> (w660:i16)
        n334 = Increment(x=w660) -> (x+1=w666:i16)
        n335 = Scale By Power Of 2(n="AI1 X Scale", x=w633) -> (x*2^n=w631:i16)
        n336 = Greater?(x=w666, y="N of AI1 Int Acq Sets") -> (0:w663:bool)
        n337 = Select(t=i16 1, s=w663, f=w666) -> (s? t:f=w665:i16)
        n338 = feedback-in #24(w665) -> ()
        n339 = Divide(x=w631, y=w634) -> (x/y=w630:fxp<+/-,16,1>)
        n340 = feedback #25(w637) -> (w635:bool)
        n341 = feedback #26(w637) -> (w653:bool)
        n342 = case shown="2" w660 {
          tunnel: w634 -> [w691 w698 _]
          tunnel: ["Set 1" "Set 2" "Set 3"] -> w658
          tunnel: ["AI to FIFO" w700 w705] -> w652
          tunnel: w653 -> [_ w700 w705]
          tunnel: ["Trap Pos to FIFO" w699 w704] -> w636
          tunnel: w635 -> [_ w699 w704]
          tunnel: w630 -> [w690 w697 _]
          tunnel: [w689 w695 FALSE] -> w617
          tunnel: [w688 w696 u64 0 ("BD1 Frequency Out 2")] -> w616
          frame 1, Default {
            n343 = local read "BD1 Frequency Out 1"() -> (w688:u64)
            n344 = Compound Arithmetic op=AND("Trap Pos to FIFO", "Set 1", "AI to FIFO") -> (w689:bool)
            "AI2 Y Sum Set 1" <- w691
            "AI1 X Set 1" <- w690
          }
          frame 2 {
            n345 = local read "BD1 Frequency Out 2"() -> (w696:u64)
            n346 = Compound Arithmetic op=AND(w699, "Set 2", w700) -> (w695:bool)
            "AI2 Y Sum Set 2" <- w698
            "AI1 X Set 2" <- w697
          }
          frame 3 {
          }
        }
        n347 = And(x=w658, y=w652) -> (x .and. y?=w659:bool)
        n348 = case shown="True" w659 {
          tunnel: w668 -> [_ w719]
          tunnel: w633 -> [_ w718]
          tunnel: w634 -> [_ w717]
          tunnel: w667 -> [_ w716]
          tunnel: w657 -> [_ w715]
          tunnel: w656 -> [_ w714]
          tunnel: w655 -> [_ w713]
          tunnel: w654 -> [_ w712]
          tunnel: 0 ("DMA buffer timeout") -> [_ w721]
          frame False {
          }
          frame True {
            n349 = Build Array(w719, w718, w717, w716, w715, w714, w713, w712) -> (w720:i16[])
            n350 = for {
              tunnel: w720 -> [w723] mode=indexing
              tunnel: w721 -> [w724]
              tunnel: [w722] -> w710 mode=indexing
              n351 = xnode ("FIFO Write")("Element"=w723, "Timeout"=w724) -> ("Timed Out?"=w722:bool)  [unwired: 1 in, 1 out]
            }
            n352 = Or Array Elements(Boolean array=w710) -> (logical OR=w707:bool)
            n353 = Boolean To (0,1)(Boolean=w707) -> (0, 1=w709:i16)
            n354 = feedback #27(u16 0) -> (w708:u16)
            n355 = Add(x=w709, y=w708) -> (x+y=w706:u16)
            "Trap AI FIFO Timeout" <- w706
            n356 = feedback-in #27(w706) -> ()
          }
        }
        n357 = feedback-in #25(w636) -> ()
        n358 = feedback-in #26(w652) -> ()
        n359 = case shown="True" w617 {
          tunnel: w616 -> [_ w674]
          tunnel: [u8 0 w671] -> w615
          frame False {
          }
          frame True {
            n360 = Split Number(x=w674) -> (hi(x)=w675:u32, lo(x)=w676:u32)
            n361 = Split Number(x=w675) -> (lo(x)=w677:u16)  [unwired: 1 out]
            n362 = Split Number(x=w676) -> (hi(x)=w678:u16, lo(x)=w679:u16)
            n363 = Build Array "BD 1 nu Stack"(w677, w678, w679) -> (w673:u16[])
            n364 = for {
              tunnel: w673 -> [w686] mode=indexing
              shift-right: [w682] -> w671
              shift-left: u8 0 -> [w683]
              n365 = xnode ("FIFO Method Node")("Element"=w686, "Timeout"="Trap FIFO Set Timeout") -> ("Timed Out?"=w685:bool)  [unwired: 1 in, 1 out]
              n366 = Boolean To (0,1)(Boolean=w685) -> (0, 1=w684:i16)
              n367 = To Unsigned Byte Integer(number=w684) -> (unsigned 8bit integer=w681:u8)
              n368 = Add(x=w681, y=w683) -> (x+y=w682:u8)
            }
          }
        }
        n369 = To Unsigned Word Integer(number=w615) -> (unsigned 16bit integer=w614:u16)
        n370 = feedback #28(u16 0) -> (w628:u16)
        n371 = Add(x=w614, y=w628) -> (x+y=w627:u16)
        "Trap Pos FIFO Timeout" <- w627
        n372 = feedback-in #28(w627) -> ()
        n373 = feedback-in #29(w651) -> ()
        n374 = feedback #29(w651) -> (w650:u16)
        n375 = Subtract(x=w651, y=w650) -> (x-y=w649:u16)
        n376 = xnode "FPGA I/O Node"("Connector1/DIO31"=FALSE ("Connector1/DIO34")) -> ()  [unwired: 1 in, 1 out]
        n377 = Subtract(x=w649, y=w648) -> (x-y=w619:u16)
        n378 = Boolean To (0,1)(Boolean="+ phase") -> (0, 1=w644:i16)
        n379 = Multiply(x=w644, y="Phase count adjustment") -> (x*y=w638:i16)
        n380 = Subtract(x="ai count", y=w619) -> (x-y=w642:u16)
        n381 = Number To Boolean Array(number=w619) -> (Boolean array=w620:bool[])
        n382 = feedback #30(i16 0) -> (w640:i16)
        n383 = Add(x=w642, y=w638) -> (x+y=w641:u16)
        n384 = Subtract(x=w640, y=w638) -> (x-y=w639:i16)
        "Relative phase" <- w639
        n385 = feedback-in #30(w639) -> ()
        n386 = Or Array Elements(Boolean array=w620) -> (logical OR=w618:bool)
        n387 = Boolean To (0,1)(Boolean=w618) -> (0, 1=w625:i16)
        n388 = To Unsigned Byte Integer(number=w625) -> (unsigned 8bit integer=w622:u8)
        n389 = feedback #31(u8 0) -> (w623:u8)
        n390 = Add(x=w622, y=w623) -> (x+y=w621:u8)
        "AI Late Counter" <- w621
        n391 = feedback-in #31(w621) -> ()
      }
    }
  }
  n392 = while "Green and red fluorescent laser interlacing (Current AO to IA 532 nm AOM ME amp)." {
    shift-right: [w733] -> _
    shift-left: w1 -> [w736]
    shift-right: [w730] -> _
    shift-left: w3 -> [w728]
    shift-right: [w727] -> _
    shift-left: w3 -> [w726]
    stop <- FALSE stop-if-true
    n393 = flat-sequence {
      tunnel: w736 -> [w740]
      tunnel: [w741] -> w735
      tunnel: [w740] -> w734
      tunnel: [w739] -> w729
      tunnel: w728 -> [w739]
      tunnel: w726 -> [w738]
      tunnel: [w738] -> w725
      tunnel: [w745] -> w732
      tunnel: w735 -> [w745]
      tunnel: [w744] -> w731
      tunnel: w734 -> [w744]
      tunnel: w729 -> [w743]
      tunnel: w725 -> [w742]
      tunnel: [w766] -> w733
      tunnel: [w782] -> w730
      tunnel: w732 -> [w793]
      tunnel: w731 -> [w790]
      tunnel: [w750] -> w727
      frame #0 {
        n394 = call "Loop Timer10"("Count(Ticks)"=w740) -> ("Tick Count(Ticks)"=w741:u16)
      }
      frame #1 {
        n395 = xnode "FPGA I/O Node"("Chassis2/Mod4/AO0"=w743, "Chassis2/Mod4/AO1"=w742) -> ()  [unwired: 2 in, 2 out]
      }
      frame #2 {
        # "Design note:\n\nThese two laser controls are in the same loop\nbecause the expansion current AI cannot separately\ntime the outputs fast enough for us.  Apparently\nit is because of communication time between the\nexpansion card and the fpga.\n\nSo the two analog control signals have the same timing\nand profile, but independent amplitudes to independently\ncontrol the intensity and feedback for each laser."
        n396 = feedback #32(TRUE) -> (w746:bool)
        n397 = Not(x=w746) -> (.not. x?=w747:bool)
        n398 = feedback-in #32(w747) -> ()
        n399 = Subtract(x="Green interlace OFF count 2", y="Green int current ON count adj") -> (x-y=w775:u16)
        n400 = feedback-in #33(w793) -> ()
        n401 = feedback #33(w793) -> (w792:u16)
        n402 = Add(x="Green int current ON count adj", y="Green interlace ON count 2") -> (x+y=w776:u16)
        n403 = Subtract(x=w793, y=w792) -> (x-y=w791:u16)
        n404 = Select(t=w776, s=w747, f=w775) -> (s? t:f=w787:u16)
        n405 = Subtract(x=w791, y=w790) -> (x-y=w759:u16)
        n406 = case shown="2" "RI Operating Mode 2" {
          tunnel: [TRUE FALSE w799] -> w748
          tunnel: w746 -> [_ _ w796]
          frame 0, Default {
          }
          frame 1 {
          }
          frame 2 {
            n407 = Not(x=w796) -> (.not. x?=w798:bool)
            n408 = Select(t=w798, s="Invert RI 2", f=w796) -> (s? t:f=w799:bool)
          }
        }
        n409 = Subtract(x=w787, y=w759) -> (x-y=w770:u16)
        n410 = case shown="0, Default" "Operating Mode 2" {
          tunnel: [TRUE FALSE w833] -> w751
          tunnel: w746 -> [_ _ w830]
          frame 0, Default {
          }
          frame 1 {
          }
          frame 2 {
            n411 = Not(x=w830) -> (.not. x?=w832:bool)
            n412 = Select(t=w832, s="Invert GI 2", f=w830) -> (s? t:f=w833:bool)
          }
        }
        n413 = Number To Boolean Array(number=w759) -> (Boolean array=w760:bool[])
        n414 = Boolean To (0,1)(Boolean="+ phase (GI) 2") -> (0, 1=w772:i16)
        n415 = Or Array Elements(Boolean array=w760) -> (logical OR=w758:bool)
        n416 = Boolean To (0,1)(Boolean=w758) -> (0, 1=w765:i16)
        n417 = Multiply(x=w772, y="Phase count adjustment (GI) 2") -> (x*y=w768:i16)
        n418 = To Unsigned Byte Integer(number=w765) -> (unsigned 8bit integer=w761:u8)
        n419 = Add(x=w770, y=w768) -> (x+y=w766:u16)
        n420 = feedback #34(u8 0) -> (w763:u8)
        n421 = Add(x=w761, y=w763) -> (x+y=w762:u8)
        "GI Late Counter 2" <- w762
        n422 = feedback-in #34(w762) -> ()
        n423 = feedback #35(i16 0) -> (w769:i16)
        n424 = Subtract(x=w769, y=w768) -> (x-y=w767:i16)
        "GI Relative phase 2" <- w767
        n425 = feedback-in #35(w767) -> ()
        n426 = And(x=w751, y="Green FB On/Off") -> (x .and. y?=w777:bool)
        n427 = And(x=w748, y="Red FB On/Off") -> (x .and. y?=w757:bool)
        n428 = case shown="True" w777 {
          tunnel: "Current Out" -> [w814 _]
          tunnel: [w814 w823] -> w781
          frame False {
          }
          frame True {
            n429 = local read "Green FB Sum"() -> (w819:i16)
            n430 = Bundle("P3"="P3", "I3"="I3", "D3"="D3") -> (w815:cluster{"P3":i16, "I3":i16, "D3":i16})  [unwired: 1 in]
            n431 = call "Slower PID.vi"("process variable"=w819, "reset?"="Green FB Reset", "setpoint"="Green FB Setpoint", "PID gains (x 2^8)"=w815, "output range"=cluster{"output high":i16, "output low":i16} {"output high"=32767, "output low"=-32768} ("Green FB output range")) -> ("output"=w826:i16)  [unwired: 10 out]
            n432 = To Long Integer(number=w826) -> (32bit integer=w820:i32)
            n433 = Add(x=w820, y=32768) -> (x+y=w822:i32)
            n434 = To Unsigned Word Integer(number=w822) -> (unsigned 16bit integer=w823:u16)
          }
        }
        n435 = case shown="True" w757 {
          tunnel: "RI Current Out" -> [w800 _]
          tunnel: [w800 w809] -> w753
          frame False {
          }
          frame True {
            n436 = local read "Red FB Intensity"() -> (w805:i16)
            n437 = Bundle("P4"="P4", "I4"="I4", "D4"="D4") -> (w801:cluster{"P4":i16, "I4":i16, "D4":i16})  [unwired: 1 in]
            n438 = call "Slower PID.vi"("process variable"=w805, "reset?"="Red FB Reset", "setpoint"="Red FB Setpoint", "PID gains (x 2^8)"=w801, "output range"=cluster{"output high":i16, "output low":i16} {"output high"=32767, "output low"=-32768} ("Green FB output range")) -> ("output"=w812:i16)  [unwired: 10 out]
            n439 = To Long Integer(number=w812) -> (32bit integer=w806:i32)
            n440 = Add(x=w806, y=32768) -> (x+y=w808:i32)
            n441 = To Unsigned Word Integer(number=w808) -> (unsigned 16bit integer=w809:u16)
          }
        }
        n442 = Boolean To (0,1)(Boolean=w751) -> (0, 1=w783:i16)
        n443 = Boolean To (0,1)(Boolean=w748) -> (0, 1=w752:i16)
        n444 = To Unsigned Word Integer(number=w783) -> (unsigned 16bit integer=w780:u16)
        n445 = To Unsigned Word Integer(number=w752) -> (unsigned 16bit integer=w754:u16)
        n446 = Multiply(x=w780, y=w781) -> (x*y=w782:u16)
        n447 = Multiply(x=w754, y=w753) -> (x*y=w750:u16)
      }
    }
  }
  n448 = while "MCL stage control" {
    shift-right: [w846] -> _
    shift-left: w1 -> [w849]
    shift-right: [w839] -> _
    shift-left: w10 -> [w836]
    shift-right: [w838] -> _
    shift-left: w9 -> [w834]
    stop <- FALSE stop-if-true
    n449 = flat-sequence {
      tunnel: w849 -> [w853]
      tunnel: [w854] -> w845
      tunnel: [w853] -> w843
      tunnel: [w852] -> w837
      tunnel: w836 -> [w852]
      tunnel: [w851] -> w835
      tunnel: w834 -> [w851]
      tunnel: w845 -> [w858]
      tunnel: [w858] -> w844
      tunnel: w843 -> [w857]
      tunnel: [w857] -> w842
      tunnel: w837 -> [w856]
      tunnel: w835 -> [w855]
      tunnel: w844 -> [w866]
      tunnel: w842 -> [w865]
      tunnel: [w866] -> w848
      tunnel: [w865] -> w847
      tunnel: [w864] -> w841
      tunnel: [w863] -> w840
      tunnel: [w938] -> w846
      tunnel: w848 -> [w945]
      tunnel: w847 -> [w942]
      tunnel: w841 -> [w940]
      tunnel: w840 -> [w939]
      tunnel: [w940] -> w839
      tunnel: [w939] -> w838
      frame #0 {
        n450 = call "Loop Timer5"("Count(Ticks)"=w853) -> ("Tick Count(Ticks)"=w854:u32)
      }
      frame #1 {
        n451 = xnode "FPGA I/O Node"("Connector0/AO1"=w856, "Connector0/AO2"=w855) -> ()  [unwired: 2 in, 2 out]
      }
      frame #2 {
        n452 = local read "Scanning MCL"() -> (w878:bool)
        n453 = Or(x=w878, y="Start scan (MCL)") -> (x .or. y?=w873:bool)
        n454 = Not(x="Abort scan (MCL)") -> (.not. x?=w871:bool)
        n455 = And(x=w871, y=w873) -> (x .and. y?=w870:bool)
        n456 = case "Raster scan" shown="True" w870 {
          tunnel: [w879 w922] -> w875
          tunnel: "Start scan (MCL)" -> [_ w907]
          tunnel: [w879 w883] -> w859
          frame False {
            w879 = i16 0
            n457 = local write "Scanning MCL"(FALSE ("scanning")) -> ()
          }
          frame True {
            w893 = i16 0
            w892 = u64 0
            # "scan incr."
            # "freq. incr. mult."
            # "count steps"
            # "count number of cycles"
            n458 = feedback #36(w892) -> (w919:u64)
            n459 = Select(t=w892, s=w907, f=w919) -> (s? t:f=w921:u64)
            n460 = Increment(x=w921) -> (x+1=w918:u64)
            n461 = Greater?(x="Cycles per step (MCL)", y=w918) -> (0:w902:bool)
            n462 = Select(t=w918, s=w902, f=w892) -> (s? t:f=w917:u64)
            n463 = feedback-in #36(w917) -> ()
            n464 = feedback #37(w892) -> (w916:u64)
            n465 = Select(t=w892, s=w907, f=w916) -> (s? t:f=w911:u64)
            n466 = Increment(x=w911) -> (x+1=w915:u64)
            n467 = Add(x="Scan steps (MCL)", y="Scan steps (MCL)") -> (x+y=w914:u64)
            n468 = Select(t=w911, s=w902, f=w915) -> (s? t:f=w897:u64)
            n469 = Greater?(x=w914, y=w897) -> (0:w896:bool)
            n470 = Select(t=w897, s=w896, f=w892) -> (s? t:f=w912:u64)
            n471 = feedback-in #37(w912) -> ()
            n472 = Equal?(x="Scan steps (MCL)", y=w897) -> (x = y?=w901:bool)
            n473 = Greater?(x="Scan steps (MCL)", y=w911) -> (0:w910:bool)
            n474 = feedback #38(w893) -> (w913:i16)
            n475 = Select(t=w893, s=w907, f=w913) -> (s? t:f=w899:i16)
            n476 = Increment(x=w899) -> (x+1=w909:i16)
            n477 = Decrement(x=w899) -> (x-1=w908:i16)
            n478 = Select(t=w909, s=w910, f=w908) -> (s? t:f=w900:i16)
            n479 = Select(t=w899, s=w901, f=w900) -> (s? t:f=w898:i16)
            n480 = Select(t=w899, s=w902, f=w898) -> (s? t:f=w894:i16)
            n481 = Select(t=w894, s=w896, f=w893) -> (s? t:f=w895:i16)
            n482 = feedback-in #38(w895) -> ()
            n483 = feedback #39(w892) -> (w906:u64)
            n484 = Select(t=w892, s=w907, f=w906) -> (s? t:f=w881:u64)
            n485 = Increment(x=w881) -> (x+1=w903:u64)
            n486 = Select(t=w881, s=w896, f=w903) -> (s? t:f=w882:u64)
            n487 = Greater?(x="Number of scans (MCL)", y=w882) -> (0:w889:bool)
            n488 = Multiply(x="Scan freq.  increment (MCL)", y=w899) -> (x*y=w922:i16)
            n489 = Select(t=TRUE, s="Cont. Scan (MCL)", f=w889) -> (s? t:f=w888:bool)
            "Scanning MCL" <- w888
            n490 = Select(t=w882, s=w888, f=w892) -> (s? t:f=w904:u64)
            n491 = feedback-in #39(w904) -> ()
            n492 = Increment(x=w882) -> (x+1=→"Scan I (MCL)":u64)
            n493 = To Word Integer(number=w881) -> (16bit integer=w884:i16)
            n494 = Multiply(x=w884, y="Scan freq.  increment (MCL)") -> (x*y=w883:i16)
          }
        }
        n495 = Select(t=w859, s="1D or 2D Scan?", f=i16 0) -> (s? t:f=w860:i16)
        n496 = Select(t=w860, s="MCL Scan Axis", f=w875) -> (s? t:f=w874:i16)
        n497 = Select(t=w875, s="MCL Scan Axis", f=w860) -> (s? t:f=w876:i16)
        n498 = Add(x=w874, y="AO2") -> (x+y=w863:i16)
        n499 = Add(x="AO1", y=w876) -> (x+y=w864:i16)
      }
      frame #3 {
        n500 = feedback-in #40(w945) -> ()
        n501 = feedback #40(w945) -> (w944:u32)
        n502 = Boolean To (0,1)(Boolean="+ phase (MCL)") -> (0, 1=w936:i16)
        n503 = Subtract(x=w945, y=w944) -> (x-y=w943:u32)
        n504 = Multiply(x=w936, y="Phase count adjustment (MCL)") -> (x*y=w932:i16)
        n505 = Subtract(x=w943, y=w942) -> (x-y=w924:u32)
        n506 = Subtract(x="MCL count", y=w924) -> (x-y=w934:u32)
        n507 = feedback #41(i16 0) -> (w933:i16)
        n508 = Subtract(x=w933, y=w932) -> (x-y=w931:i16)
        "MCL Relative Phase" <- w931
        n509 = feedback-in #41(w931) -> ()
        n510 = Number To Boolean Array(number=w924) -> (Boolean array=w925:bool[])
        n511 = Or Array Elements(Boolean array=w925) -> (logical OR=w923:bool)
        n512 = Boolean To (0,1)(Boolean=w923) -> (0, 1=w930:i16)
        n513 = Add(x=w934, y=w932) -> (x+y=w938:u32)
        n514 = To Unsigned Byte Integer(number=w930) -> (unsigned 8bit integer=w927:u8)
        n515 = feedback #42(u8 0) -> (w928:u8)
        n516 = Add(x=w927, y=w928) -> (x+y=w926:u8)
        "MCL Late Counter" <- w926
        n517 = feedback-in #42(w926) -> ()
      }
    }
  }
  n518 = while "Excitation laser intensity feedback measurement (all lasers)" {
    shift-right: [w947] -> _
    shift-left: w1 -> [w952]
    stop <- FALSE stop-if-true
    n519 = flat-sequence {
      tunnel: w952 -> [w954]
      tunnel: [w955] -> w950
      tunnel: [w954] -> w948
      tunnel: [w961] -> w951
      tunnel: w950 -> [w961]
      tunnel: [w960] -> w949
      tunnel: w948 -> [w960]
      tunnel: [w973] -> w947
      tunnel: w951 -> [w984]
      tunnel: w949 -> [w981]
      frame #0 {
        n520 = call "Loop Timer9"("Count(Ticks)"=w954) -> ("Tick Count(Ticks)"=w955:u16)
      }
      frame #1 {
        # "Design note:\n\nAll lasers need to be measured at the same \ntime because the AI expansion module\ncannot independently time the measurements\nwithin our requirements: their is dead time.\n\nThis probably wouldn't be an issue with the built\nin AI on the fpga board itself."
        n521 = xnode "FPGA I/O Node"("Connector1/DIO35"=TRUE) -> ("Chassis2/Mod1/AI2"=→"Blue Intensity":i16, "Chassis2/Mod1/AI1"=→"Red FB Intensity":i16, "Chassis2/Mod1/AI0"=→"Green FB Sum":i16)  [unwired: 4 in, 4 out]
      }
      frame #2 {
        n522 = feedback-in #43(w984) -> ()
        n523 = feedback #43(w984) -> (w983:u16)
        n524 = Subtract(x=w984, y=w983) -> (x-y=w982:u16)
        n525 = xnode "FPGA I/O Node"("Connector1/DIO35"=FALSE) -> ()  [unwired: 1 in, 1 out]
        n526 = Subtract(x=w982, y=w981) -> (x-y=w963:u16)
        n527 = Subtract(x="Green FB Count", y=w963) -> (x-y=w977:u16)
        n528 = Number To Boolean Array(number=w963) -> (Boolean array=w964:bool[])
        n529 = Or Array Elements(Boolean array=w964) -> (logical OR=w962:bool)
        n530 = Boolean To (0,1)(Boolean="+ phase (Green FB)") -> (0, 1=w975:i16)
        n531 = Boolean To (0,1)(Boolean=w962) -> (0, 1=w969:i16)
        n532 = Multiply(x=w975, y="Phase count adjustment (Green FB)") -> (x*y=w970:i16)
        n533 = Add(x=w977, y=w970) -> (x+y=w973:u16)
        n534 = To Unsigned Byte Integer(number=w969) -> (unsigned 8bit integer=w966:u8)
        n535 = feedback #44(i16 0) -> (w972:i16)
        n536 = Subtract(x=w972, y=w970) -> (x-y=w971:i16)
        "Green FB Relative Phase" <- w971
        n537 = feedback-in #44(w971) -> ()
        n538 = feedback #45(u8 0) -> (w967:u8)
        n539 = Add(x=w966, y=w967) -> (x+y=w965:u8)
        "Green Late Counter" <- w965
        n540 = feedback-in #45(w965) -> ()
      }
    }
  }
  n541 = while "APD 1 Gating" {
    shift-right: [w988] -> _
    shift-left: w1 -> [w993]
    shift-right: [w987] -> _
    shift-left: w5 -> [w985]
    stop <- FALSE stop-if-true
    n542 = flat-sequence {
      tunnel: w993 -> [w996]
      tunnel: [w997] -> w991
      tunnel: [w996] -> w989
      tunnel: [w995] -> w986
      tunnel: w985 -> [w995]
      tunnel: [w1000] -> w992
      tunnel: w991 -> [w1000]
      tunnel: [w999] -> w990
      tunnel: w989 -> [w999]
      tunnel: w986 -> [w998]
      tunnel: [w1014] -> w988
      tunnel: w992 -> [w1029]
      tunnel: w990 -> [w1026]
      tunnel: [w1018] -> w987
      frame #0 {
        n543 = call "Loop Timer7"("Count(Ticks)"=w996) -> ("Tick Count(Ticks)"=w997:u16)
      }
      frame #1 {
        # "Signal is then sent through \na transistor before APD"
        n544 = xnode "FPGA I/O Node"("Connector0/DIO4"=w998) -> ()  [unwired: 1 in, 1 out]
      }
      frame #2 {
        n545 = feedback #46(TRUE) -> (w1021:bool)
        n546 = feedback-in #47(w1029) -> ()
        n547 = feedback #47(w1029) -> (w1028:u16)
        n548 = Not(x=w1021) -> (.not. x?=w1017:bool)
        n549 = feedback-in #46(w1017) -> ()
        n550 = Subtract(x=w1029, y=w1028) -> (x-y=w1027:u16)
        n551 = Select(t="APD Gate ON Count", s=w1017, f="APD Gate OFF Count") -> (s? t:f=w1023:u16)
        n552 = Subtract(x=w1027, y=w1026) -> (x-y=w1002:u16)
        n553 = Subtract(x=w1023, y=w1002) -> (x-y=w1013:u16)
        n554 = Number To Boolean Array(number=w1002) -> (Boolean array=w1003:bool[])
        n555 = Or Array Elements(Boolean array=w1003) -> (logical OR=w1001:bool)
        n556 = Boolean To (0,1)(Boolean="+ phase (APD 1 Gate)") -> (0, 1=w1011:i16)
        n557 = Boolean To (0,1)(Boolean=w1001) -> (0, 1=w1008:i16)
        n558 = Multiply(x=w1011, y="Phase count adjustment (APD 1 Gate)") -> (x*y=w1009:i16)
        n559 = To Unsigned Byte Integer(number=w1008) -> (unsigned 8bit integer=w1005:u8)
        n560 = Add(x=w1013, y=w1009) -> (x+y=w1014:u16)
        n561 = feedback #48(i16 0) -> (w1016:i16)
        n562 = Subtract(x=w1016, y=w1009) -> (x-y=w1015:i16)
        "APD 1 Gate Relative Phase" <- w1015
        n563 = feedback-in #48(w1015) -> ()
        n564 = feedback #49(u8 0) -> (w1006:u8)
        n565 = Add(x=w1005, y=w1006) -> (x+y=w1004:u8)
        "APD 1 Gate Late Counter" <- w1004
        n566 = feedback-in #49(w1004) -> ()
        n567 = case shown="2" "APD Gate Operating Mode" {
          tunnel: [TRUE FALSE w1035] -> w1018
          tunnel: w1021 -> [_ _ w1032]
          frame 0, Default {
          }
          frame 1 {
          }
          frame 2 {
            n568 = Not(x=w1032) -> (.not. x?=w1034:bool)
            n569 = Select(t=w1034, s="Invert APD Gate", f=w1032) -> (s? t:f=w1035:bool)
          }
        }
      }
    }
  }
  n570 = while "Control APD data integration - stream to host" {
    shift-right: [w1039] -> _
    shift-left: w6 -> [w1044]
    stop <- FALSE stop-if-true
    n571 = flat-sequence {
      tunnel: w1044 -> [w1046]
      tunnel: [w1047] -> w1042
      tunnel: [w1046] -> w1040
      tunnel: [w1057] -> w1043
      tunnel: w1042 -> [w1057]
      tunnel: [w1056] -> w1041
      tunnel: w1040 -> [w1056]
      tunnel: [w1055] -> w1038
      tunnel: [w1054] -> w1037
      tunnel: [w1048] -> w1036
      tunnel: [w1099] -> w1039
      tunnel: w1043 -> [w1109]
      tunnel: w1041 -> [w1106]
      tunnel: w1038 -> [w1092]
      tunnel: w1037 -> [w1091]
      tunnel: w1036 -> [w1079]
      frame #0 {
        n572 = call "Loop Timer6"("Count(Ticks)"=w1046) -> ("Tick Count(Ticks)"=w1047:u32)
      }
      frame #1 {
        n573 = flat-sequence {
          tunnel: [w1059] -> w1053
          tunnel: w1053 -> [w1062]
          tunnel: [w1066] -> w1052
          tunnel: [w1065] -> w1051
          tunnel: [w1062] -> w1050
          tunnel: [w1061] -> w1049
          tunnel: [w1073] -> w1054
          tunnel: [w1074] -> w1055
          tunnel: w1052 -> [w1074]
          tunnel: w1051 -> [w1073]
          tunnel: w1050 -> [w1072]
          tunnel: w1049 -> [w1071]
          tunnel: [w1071] -> w1048
          frame #0 {
            # "use separate variable so each APD won't\nhave to wait to read"
            n574 = feedback #50(FALSE) -> (w1058:bool)
            "APD1 out state" <- w1058
            "APD2 out state" <- w1058
            "APD3 out state" <- w1058
            n575 = Not(x=w1058) -> (.not. x?=w1059:bool)
            n576 = feedback-in #50(w1059) -> ()
          }
          frame #1 {
            n577 = local read "APD 3 Counts 1"() -> (w1064:u32)
            n578 = local read "APD 3 Counts 0"() -> (w1063:u32)
            n579 = local read "APD 1 Counts 1"() -> (w1070:u32)
            n580 = local read "APD 1 Counts 0"() -> (w1069:u32)
            n581 = local read "APD 2 Counts 1"() -> (w1068:u32)
            n582 = local read "APD 2 Counts 0"() -> (w1067:u32)
            n583 = Select(t=w1064, s=w1062, f=w1063) -> (s? t:f=w1061:u32)
            n584 = Select(t=w1070, s=w1062, f=w1069) -> (s? t:f=w1066:u32)
            n585 = Select(t=w1068, s=w1062, f=w1067) -> (s? t:f=w1065:u32)
          }
          frame #2 {
            n586 = case shown="False" w1072 {
              frame False {
                w1075 = u32 0 ("APD 1 Counts 0")
                n587 = local write "APD 1 Counts 0"(w1075) -> ()
                n588 = local write "APD 2 Counts 0"(w1075) -> ()
                n589 = local write "APD 3 Counts 0"(w1075) -> ()
              }
              frame True {
                w1076 = u32 0 ("APD 1 Counts 1")
                n590 = local write "APD 1 Counts 1"(w1076) -> ()
                n591 = local write "APD 2 Counts 1"(w1076) -> ()
                n592 = local write "APD 3 Counts 1"(w1076) -> ()
              }
            }
          }
        }
      }
      frame #2 {
        n593 = feedback-in #51(w1109) -> ()
        n594 = feedback #51(w1109) -> (w1108:u32)
        n595 = Subtract(x=w1109, y=w1108) -> (x-y=w1107:u32)
        n596 = Subtract(x=w1107, y=w1106) -> (x-y=w1084:u32)
        n597 = case shown="True" "APD to FIFO" {
          tunnel: w1092 -> [_ w1114]
          tunnel: w1091 -> [_ w1112]
          tunnel: w1079 -> [_ w1110]
          frame False {
          }
          frame True {
            n598 = flat-sequence {
              tunnel: 0 ("Timeout") -> [w1116]
              tunnel: w1114 -> [w1117]
              tunnel: [w1116] -> w1113
              tunnel: w1113 -> [w1118]
              tunnel: w1112 -> [w1119]
              tunnel: [w1118] -> w1111
              tunnel: w1111 -> [w1121]
              tunnel: w1110 -> [w1120]
              frame #0 {
                n599 = xnode ("FIFO Write")("Element"=w1117, "Timeout"=w1116) -> ()  [unwired: 1 in, 2 out]
              }
              frame #1 {
                n600 = xnode ("FIFO Write")("Element"=w1119, "Timeout"=w1118) -> ()  [unwired: 1 in, 2 out]
              }
              frame #2 {
                n601 = xnode ("FIFO Write")("Element"=w1120, "Timeout"=w1121) -> ()  [unwired: 1 in, 2 out]
              }
            }
          }
        }
        n602 = Subtract(x="APD Acq Rate Count", y=w1084) -> (x-y=w1100:u32)
        n603 = Number To Boolean Array(number=w1084) -> (Boolean array=w1085:bool[])
        n604 = Or Array Elements(Boolean array=w1085) -> (logical OR=w1083:bool)
        n605 = Boolean To (0,1)(Boolean=w1083) -> (0, 1=w1090:i16)
        n606 = To Unsigned Byte Integer(number=w1090) -> (unsigned 8bit integer=w1087:u8)
        n607 = feedback #52(u8 0) -> (w1088:u8)
        n608 = Add(x=w1087, y=w1088) -> (x+y=w1086:u8)
        "APD Acq Late Counter" <- w1086
        n609 = feedback-in #52(w1086) -> ()
        n610 = Boolean To (0,1)(Boolean="+ phase (APD Acq)") -> (0, 1=w1096:i16)
        n611 = Multiply(x=w1096, y="Phase Count Adjustment (APD Acq)") -> (x*y=w1093:i16)
        n612 = Add(x=w1100, y=w1093) -> (x+y=w1099:u32)
        n613 = feedback #53(i16 0) -> (w1098:i16)
        n614 = Subtract(x=w1098, y=w1093) -> (x-y=w1095:i16)
        "APD Acq Relative Phase" <- w1095
        n615 = feedback-in #53(w1095) -> ()
        n616 = To Word Integer(number=w1092) -> (16bit integer=w1101:i16)
        n617 = To Word Integer(number=w1079) -> (16bit integer=w1080:i16)
        n618 = To Word Integer(number=w1091) -> (16bit integer=w1102:i16)
        n619 = Multiply(x="APD AO scale factor", y=w1102) -> (x*y=w1081:i16)
        n620 = Multiply(x="APD AO scale factor", y=w1080) -> (x*y=w1077:i16)
        n621 = Multiply(x="APD AO scale factor", y=w1101) -> (x*y=w1082:i16)
        n622 = xnode "FPGA I/O Node"("Connector0/AO5"=w1082, "Connector0/AO7"=w1081, "Connector0/AO6"=w1077) -> ()  [unwired: 3 in, 3 out]
      }
    }
  }
  n623 = node-c288(w7) -> ()
  n624 = while "APD 3 Counter" {
    tunnel: w1 -> [_]
    stop <- FALSE stop-if-true
    n625 = flat-sequence {
      frame #0 {
        n626 = xnode "FPGA I/O Method Node"("FPGA I/O In"=refnum<k21> "Connector0/DIO2" ("APD 2 DO"), "Timeout"=-1) -> ()  [unwired: 2 out]
      }
      frame #1 {
        n627 = local read "APD3 out state"() -> (w1125:bool)
        n628 = case shown="False" w1125 {
          frame False {
            n629 = local read "APD 3 Counts 0"() -> (w1127:u32)
            n630 = Increment(x=w1127) -> (x+1=→"APD 3 Counts 0":u32)
          }
          frame True {
            n631 = local read "APD 3 Counts 1"() -> (w1129:u32)
            n632 = Increment(x=w1129) -> (x+1=→"APD 3 Counts 1":u32)
          }
        }
      }
    }
  }
  n633 = while "APD 3 Gating" {
    shift-right: [w1133] -> _
    shift-left: w1 -> [w1138]
    shift-right: [w1132] -> _
    shift-left: w5 -> [w1130]
    stop <- FALSE stop-if-true
    n634 = flat-sequence {
      tunnel: w1138 -> [w1141]
      tunnel: [w1142] -> w1136
      tunnel: [w1141] -> w1134
      tunnel: [w1140] -> w1131
      tunnel: w1130 -> [w1140]
      tunnel: [w1145] -> w1137
      tunnel: w1136 -> [w1145]
      tunnel: [w1144] -> w1135
      tunnel: w1134 -> [w1144]
      tunnel: w1131 -> [w1143]
      tunnel: [w1162] -> w1133
      tunnel: w1137 -> [w1174]
      tunnel: w1135 -> [w1171]
      tunnel: [w1166] -> w1132
      frame #0 {
        n635 = call "Loop Timer15"("Count(Ticks)"=w1141) -> ("Tick Count(Ticks)"=w1142:u16)
      }
      frame #1 {
        # "Signal is then sent through \na transistor before APD"
        n636 = xnode "FPGA I/O Node"("Connector0/DIO9"=w1143) -> ()  [unwired: 1 in, 1 out]
      }
      frame #2 {
        n637 = local read "APD Gate OFF Count"() -> (w1147:u16)
        n638 = local read "APD Gate ON Count"() -> (w1148:u16)
        n639 = feedback #54(TRUE) -> (w1168:bool)
        n640 = feedback-in #55(w1174) -> ()
        n641 = feedback #55(w1174) -> (w1173:u16)
        n642 = Not(x=w1168) -> (.not. x?=w1165:bool)
        n643 = feedback-in #54(w1165) -> ()
        n644 = Subtract(x=w1174, y=w1173) -> (x-y=w1172:u16)
        n645 = Select(t=w1148, s=w1165, f=w1147) -> (s? t:f=w1170:u16)
        n646 = Subtract(x=w1172, y=w1171) -> (x-y=w1150:u16)
        n647 = Subtract(x=w1170, y=w1150) -> (x-y=w1161:u16)
        n648 = Number To Boolean Array(number=w1150) -> (Boolean array=w1151:bool[])
        n649 = Or Array Elements(Boolean array=w1151) -> (logical OR=w1149:bool)
        n650 = Boolean To (0,1)(Boolean=w1149) -> (0, 1=w1156:i16)
        n651 = Boolean To (0,1)(Boolean="+ phase (APD 3 Gate)") -> (0, 1=w1159:i16)
        n652 = To Unsigned Byte Integer(number=w1156) -> (unsigned 8bit integer=w1153:u8)
        n653 = Multiply(x=w1159, y="Phase count adjustment (APD 3 Gate)") -> (x*y=w1157:i16)
        n654 = feedback #56(u8 0) -> (w1154:u8)
        n655 = Add(x=w1153, y=w1154) -> (x+y=w1152:u8)
        "APD 3 Gate Late Counter" <- w1152
        n656 = feedback-in #56(w1152) -> ()
        n657 = Add(x=w1161, y=w1157) -> (x+y=w1162:u16)
        n658 = feedback #57(i16 0) -> (w1164:i16)
        n659 = Subtract(x=w1164, y=w1157) -> (x-y=w1163:i16)
        "APD 3 Gate Relative Phase" <- w1163
        n660 = feedback-in #57(w1163) -> ()
        n661 = local read "APD Gate Operating Mode"() -> (w1146:u8)
        n662 = case shown="2" w1146 {
          tunnel: [TRUE FALSE w1180] -> w1166
          tunnel: w1168 -> [_ _ w1178]
          frame 0, Default {
          }
          frame 1 {
          }
          frame 2 {
            n663 = local read "Invert APD Gate"() -> (w1177:bool)
            n664 = Not(x=w1178) -> (.not. x?=w1179:bool)
            n665 = Select(t=w1179, s=w1177, f=w1178) -> (s? t:f=w1180:bool)
          }
        }
      }
    }
  }
  n666 = while "633 nm red  fluorescent laser interlacing (DO to IA 633 nm AOM ME amp)." {
    shift-right: [w1184] -> _
    shift-left: w1 -> [w1189]
    shift-right: [w1183] -> _
    shift-left: w2 -> [w1181]
    stop <- FALSE stop-if-true
    n667 = flat-sequence {
      tunnel: w1189 -> [w1192]
      tunnel: [w1193] -> w1187
      tunnel: [w1192] -> w1185
      tunnel: [w1191] -> w1182
      tunnel: w1181 -> [w1191]
      tunnel: [w1196] -> w1188
      tunnel: w1187 -> [w1196]
      tunnel: [w1195] -> w1186
      tunnel: w1185 -> [w1195]
      tunnel: w1182 -> [w1194]
      tunnel: [w1205] -> w1184
      tunnel: w1188 -> [w1225]
      tunnel: w1186 -> [w1222]
      tunnel: [w1214] -> w1183
      frame #0 {
        n668 = call "Loop Timer11"("Count(Ticks)"=w1192) -> ("Tick Count(Ticks)"=w1193:u16)
      }
      frame #1 {
        # "Then to PRL 440 amp"
        n669 = xnode "FPGA I/O Node"("Connector1/DIO32"=w1194) -> ()  [unwired: 1 in, 1 out]
      }
      frame #2 {
        n670 = feedback-in #58(w1225) -> ()
        n671 = feedback #58(w1225) -> (w1224:u16)
        n672 = Subtract(x=w1225, y=w1224) -> (x-y=w1223:u16)
        n673 = Subtract(x=w1223, y=w1222) -> (x-y=w1198:u16)
        n674 = Number To Boolean Array(number=w1198) -> (Boolean array=w1199:bool[])
        n675 = Or Array Elements(Boolean array=w1199) -> (logical OR=w1197:bool)
        n676 = Boolean To (0,1)(Boolean="+ phase (RI)") -> (0, 1=w1210:i16)
        n677 = Multiply(x=w1210, y="Phase count adjustment (RI)") -> (x*y=w1207:i16)
        n678 = Boolean To (0,1)(Boolean=w1197) -> (0, 1=w1204:i16)
        n679 = To Unsigned Byte Integer(number=w1204) -> (unsigned 8bit integer=w1201:u8)
        n680 = feedback #59(i16 0) -> (w1208:i16)
        n681 = feedback #60(u8 0) -> (w1202:u8)
        n682 = Add(x=w1201, y=w1202) -> (x+y=w1200:u8)
        "RI Late Counter" <- w1200
        n683 = feedback-in #60(w1200) -> ()
        n684 = Subtract(x=w1208, y=w1207) -> (x-y=w1206:i16)
        "RI Relative phase" <- w1206
        n685 = feedback-in #59(w1206) -> ()
        n686 = feedback #61(TRUE) -> (w1217:bool)
        n687 = case shown="2" "Red Laser Operating Mode" {
          tunnel: [TRUE FALSE w1231] -> w1214
          tunnel: w1217 -> [_ _ w1228]
          frame 0, Default {
          }
          frame 1 {
          }
          frame 2 {
            n688 = Not(x=w1228) -> (.not. x?=w1230:bool)
            n689 = Select(t=w1230, s="Invert RI", f=w1228) -> (s? t:f=w1231:bool)
          }
        }
        n690 = Not(x=w1217) -> (.not. x?=w1213:bool)
        n691 = Select(t="Red interlace ON count", s=w1213, f="Red interlace OFF count") -> (s? t:f=w1219:u16)
        n692 = Subtract(x=w1219, y=w1198) -> (x-y=w1211:u16)
        n693 = Add(x=w1211, y=w1207) -> (x+y=w1205:u16)
        n694 = feedback-in #61(w1213) -> ()
      }
    }
  }
  n695 = while "473 nm blue  fluorescent laser interlacing (DO to blue laser digital control input)." {
    shift-right: [w1235] -> _
    shift-left: w1 -> [w1240]
    shift-right: [w1234] -> _
    shift-left: w2 -> [w1232]
    stop <- FALSE stop-if-true
    n696 = flat-sequence {
      tunnel: w1240 -> [w1243]
      tunnel: [w1244] -> w1238
      tunnel: [w1243] -> w1236
      tunnel: [w1242] -> w1233
      tunnel: w1232 -> [w1242]
      tunnel: [w1247] -> w1239
      tunnel: w1238 -> [w1247]
      tunnel: [w1246] -> w1237
      tunnel: w1236 -> [w1246]
      tunnel: w1233 -> [w1245]
      tunnel: [w1256] -> w1235
      tunnel: w1239 -> [w1276]
      tunnel: w1237 -> [w1273]
      tunnel: [w1265] -> w1234
      frame #0 {
        n697 = call "Loop Timer14"("Count(Ticks)"=w1243) -> ("Tick Count(Ticks)"=w1244:u16)
      }
      frame #1 {
        n698 = xnode "FPGA I/O Node"("Connector1/DIO28"=w1245) -> ()  [unwired: 1 in, 1 out]
      }
      frame #2 {
        n699 = feedback-in #62(w1276) -> ()
        n700 = feedback #62(w1276) -> (w1275:u16)
        n701 = Subtract(x=w1276, y=w1275) -> (x-y=w1274:u16)
        n702 = Subtract(x=w1274, y=w1273) -> (x-y=w1249:u16)
        n703 = Number To Boolean Array(number=w1249) -> (Boolean array=w1250:bool[])
        n704 = Or Array Elements(Boolean array=w1250) -> (logical OR=w1248:bool)
        n705 = Boolean To (0,1)(Boolean="+ phase (BI D)") -> (0, 1=w1261:i16)
        n706 = Multiply(x=w1261, y="Phase count adjustment (BI D)") -> (x*y=w1258:i16)
        n707 = Boolean To (0,1)(Boolean=w1248) -> (0, 1=w1255:i16)
        n708 = To Unsigned Byte Integer(number=w1255) -> (unsigned 8bit integer=w1252:u8)
        n709 = feedback #63(i16 0) -> (w1259:i16)
        n710 = feedback #64(u8 0) -> (w1253:u8)
        n711 = Add(x=w1252, y=w1253) -> (x+y=w1251:u8)
        "Blue Late Counter (D)" <- w1251
        n712 = feedback-in #64(w1251) -> ()
        n713 = Subtract(x=w1259, y=w1258) -> (x-y=w1257:i16)
        "BI Relative phase (D)" <- w1257
        n714 = feedback-in #63(w1257) -> ()
        n715 = feedback #65(TRUE) -> (w1268:bool)
        n716 = case shown="2" "Blue Laser Operating Mode (D)" {
          tunnel: [TRUE FALSE w1282] -> w1265
          tunnel: w1268 -> [_ _ w1279]
          frame 0, Default {
          }
          frame 1 {
          }
          frame 2 {
            n717 = Not(x=w1279) -> (.not. x?=w1281:bool)
            n718 = Select(t=w1281, s="Invert BI (D)", f=w1279) -> (s? t:f=w1282:bool)
          }
        }
        n719 = Not(x=w1268) -> (.not. x?=w1264:bool)
        n720 = Select(t="Blue interlace ON count (D)", s=w1264, f="Blue interlace OFF count (D)") -> (s? t:f=w1270:u16)
        n721 = Subtract(x=w1270, y=w1249) -> (x-y=w1262:u16)
        n722 = Add(x=w1262, y=w1258) -> (x+y=w1256:u16)
        n723 = feedback-in #65(w1264) -> ()
      }
    }
  }
  n724 = while "Blue fluorescent laser interlacing (AO control direct to laser)." {
    shift-right: [w1288] -> _
    shift-left: w1 -> [w1291]
    shift-right: [w1285] -> _
    shift-left: i16 0 -> [w1283]
    stop <- FALSE stop-if-true
    n725 = flat-sequence {
      tunnel: w1291 -> [w1294]
      tunnel: [w1295] -> w1290
      tunnel: [w1294] -> w1289
      tunnel: [w1293] -> w1284
      tunnel: w1283 -> [w1293]
      tunnel: [w1298] -> w1287
      tunnel: w1290 -> [w1298]
      tunnel: [w1297] -> w1286
      tunnel: w1289 -> [w1297]
      tunnel: w1284 -> [w1296]
      tunnel: [w1308] -> w1288
      tunnel: [w1324] -> w1285
      tunnel: w1287 -> [w1336]
      tunnel: w1286 -> [w1333]
      frame #0 {
        n726 = call "Loop Timer13"("Count(Ticks)"=w1294) -> ("Tick Count(Ticks)"=w1295:u16)
      }
      frame #1 {
        n727 = xnode "FPGA I/O Node"("Connector0/AO3"=w1296) -> ()  [unwired: 1 in, 1 out]
      }
      frame #2 {
        n728 = Subtract(x="Blue OFF count (AO)", y="Blue current ON count adj (AO)") -> (x-y=w1317:u16)
        n729 = feedback-in #66(w1336) -> ()
        n730 = feedback #66(w1336) -> (w1335:u16)
        n731 = Add(x="Blue current ON count adj (AO)", y="Blue ON count (AO)") -> (x+y=w1318:u16)
        n732 = Subtract(x=w1336, y=w1335) -> (x-y=w1334:u16)
        n733 = Subtract(x=w1334, y=w1333) -> (x-y=w1301:u16)
        n734 = Number To Boolean Array(number=w1301) -> (Boolean array=w1302:bool[])
        n735 = Boolean To (0,1)(Boolean="+ phase (BI AO)") -> (0, 1=w1314:i16)
        n736 = Or Array Elements(Boolean array=w1302) -> (logical OR=w1300:bool)
        n737 = Boolean To (0,1)(Boolean=w1300) -> (0, 1=w1307:i16)
        n738 = Multiply(x=w1314, y="Phase count adjustment (BI AO)") -> (x*y=w1310:i16)
        n739 = To Unsigned Byte Integer(number=w1307) -> (unsigned 8bit integer=w1303:u8)
        n740 = feedback #67(u8 0) -> (w1305:u8)
        n741 = Add(x=w1303, y=w1305) -> (x+y=w1304:u8)
        "BI Late Counter (AO)" <- w1304
        n742 = feedback-in #67(w1304) -> ()
        n743 = feedback #68(i16 0) -> (w1311:i16)
        n744 = Subtract(x=w1311, y=w1310) -> (x-y=w1309:i16)
        "BI Relative phase (AO)" <- w1309
        n745 = feedback-in #68(w1309) -> ()
        n746 = feedback #69(TRUE) -> (w1328:bool)
        n747 = case shown="2" "BI Operating Mode (AO)" {
          tunnel: [TRUE FALSE w1352] -> w1319
          tunnel: w1328 -> [_ _ w1349]
          frame 0, Default {
          }
          frame 1 {
          }
          frame 2 {
            n748 = Not(x=w1349) -> (.not. x?=w1351:bool)
            n749 = Select(t=w1351, s="Invert BI (AO)", f=w1349) -> (s? t:f=w1352:bool)
          }
        }
        n750 = And(x=w1319, y="Blue FB On/Off") -> (x .and. y?=w1320:bool)
        n751 = case shown="True" w1320 {
          tunnel: "BI Current Out" -> [w1337 _]
          tunnel: [w1337 w1339] -> w1323
          frame False {
          }
          frame True {
            n752 = local read "Blue Intensity"() -> (w1338:i16)
            n753 = Bundle("P5"="P5", "I5"="I5", "D5"="D5") -> (w1340:cluster{"P5":i16, "I5":i16, "D5":i16})  [unwired: 1 in]
            n754 = call "Slower PID.vi"("process variable"=w1338, "reset?"="Blue FB Reset", "setpoint"="Blue FB Setpoint", "PID gains (x 2^8)"=w1340, "output range"=cluster{"output high":i16, "output low":i16} {"output high"=32767, "output low"=0} ("Green FB output range")) -> ("output"=w1339:i16)  [unwired: 10 out]
          }
        }
        n755 = Not(x=w1328) -> (.not. x?=w1325:bool)
        n756 = Select(t=w1318, s=w1325, f=w1317) -> (s? t:f=w1330:u16)
        n757 = Subtract(x=w1330, y=w1301) -> (x-y=w1312:u16)
        n758 = Add(x=w1312, y=w1310) -> (x+y=w1308:u16)
        n759 = feedback-in #69(w1325) -> ()
        n760 = Boolean To (0,1)(Boolean=w1319) -> (0, 1=w1299:i16)
        n761 = Multiply(x=w1299, y=w1323) -> (x*y=w1324:i16)
      }
    }
  }
